vi "HandleObservationAsync.vi"(8 "error in (no error)":errorcluster, 10 "Acquisition.lvclass In":refnum<class "Acquisition.lvclass">, 11 "S4ACS_GUI in":refnum<class "S4GUI.lvclass">) -> (0 "error out":errorcluster, 2 "Acquisition.lvclass Out":refnum<class "Acquisition.lvclass">, 3 "S4ACS_GUI out":refnum<class "S4GUI.lvclass">)   [LabVIEW 2018, in "S4GUI.lvclass"]
uses:
  S4GUI.lvclass
  Acquisition/Acquisition.lvclass
  S4GUI.lvclass/S4GUI.ctl
  Instrument/Instrument.lvclass/Instrument.ctl
  Device/Optics/Optics.lvclass/Optics.ctl
  Server/Server.lvclass/Server.ctl
  Device/Optics/Opt_Selector/Opt_Selector.lvclass
  C:/Users/observer/Desktop/Sparc4GUI/SPARC4_GUI/Device/Optics/Optics.lvclass
  SyncBox/Sync Box.lvclass
  C:/Users/observer/Desktop/Sparc4GUI/SPARC4_GUI/Server/Server.lvclass
  Instrument/Instrument.lvclass
  StateMachine/State Machine.lvclass
  Trigger/Trigger.lvclass
  Channel/Channel.lvclass
  Device/Optics/Optics.lvclass
  Server/Server.lvclass
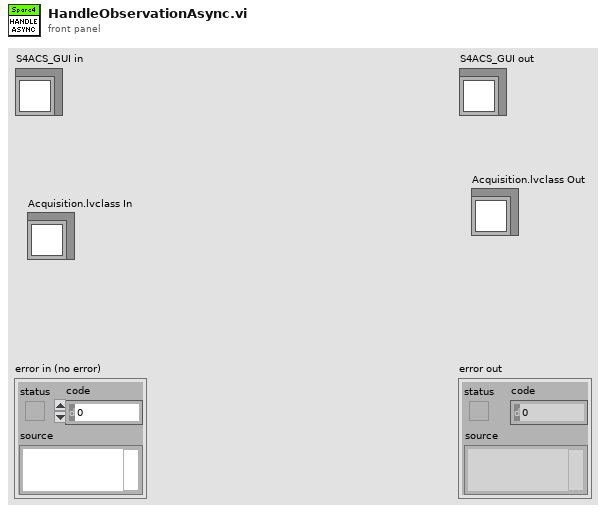
[diagram p1: front panel]
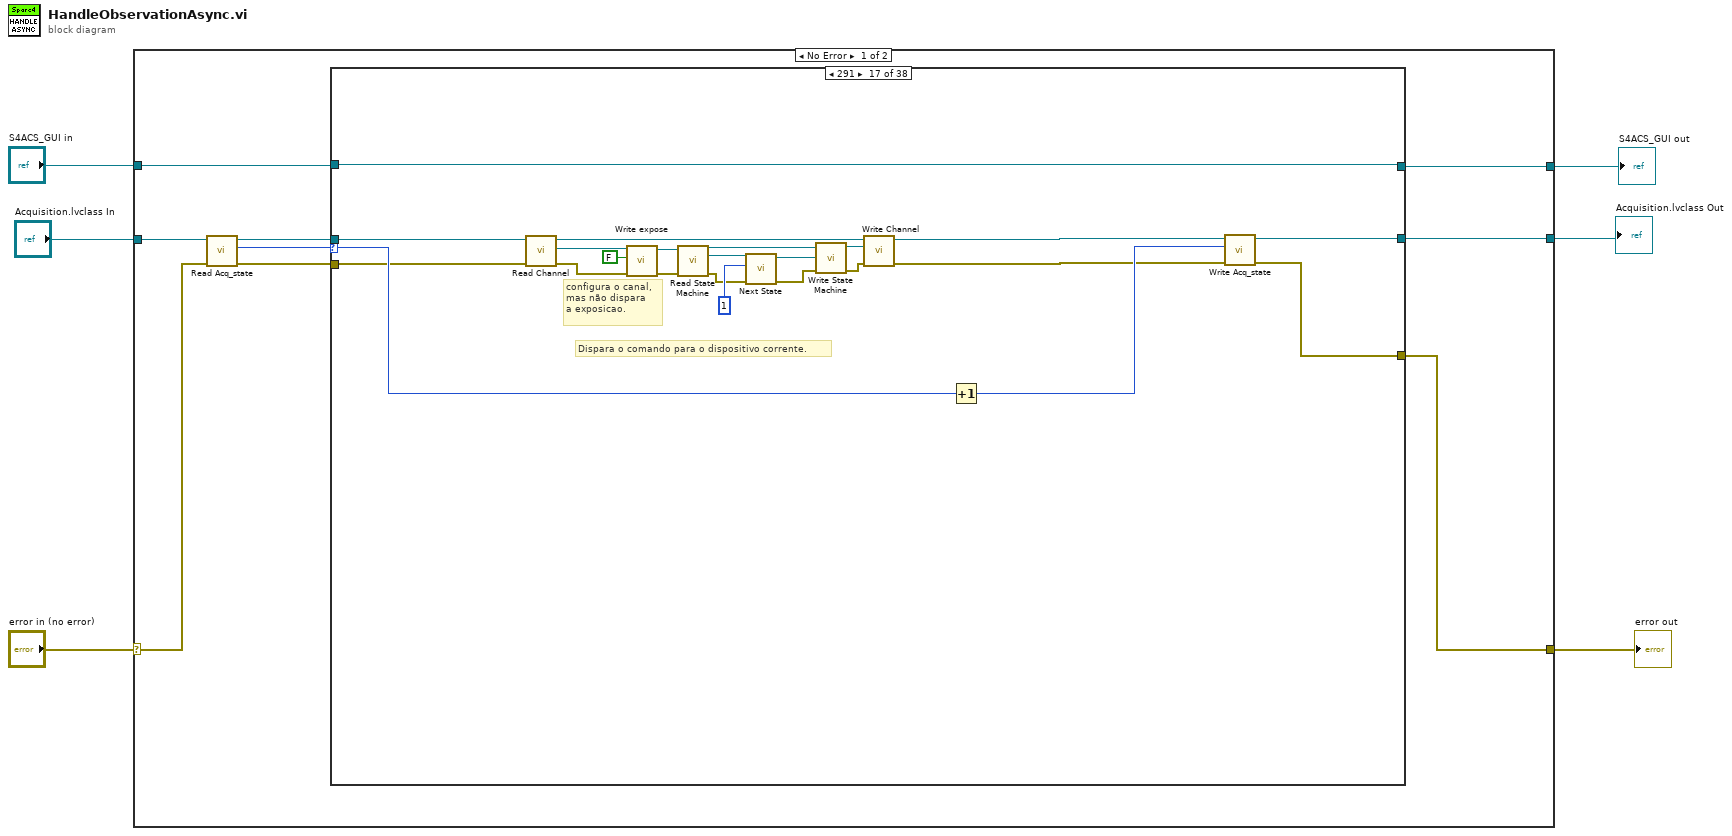
[diagram p0: block diagram]
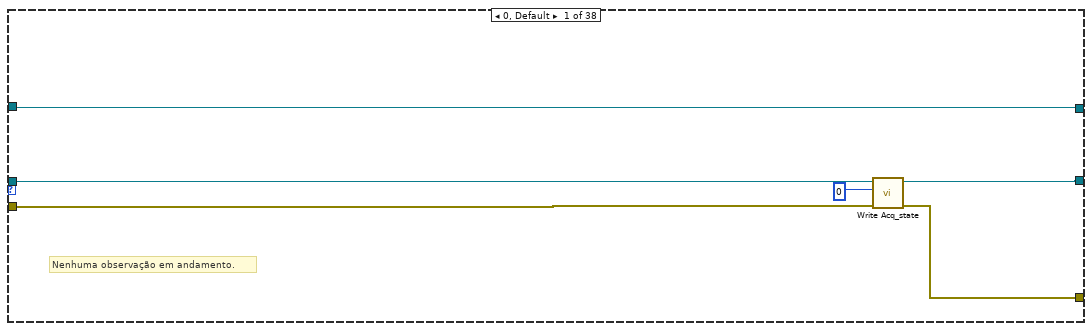
[diagram p2: hidden frame]
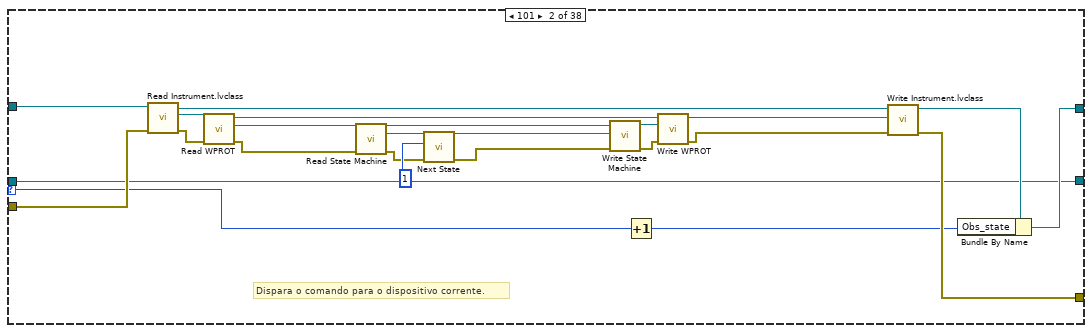
[diagram p3: hidden frame]
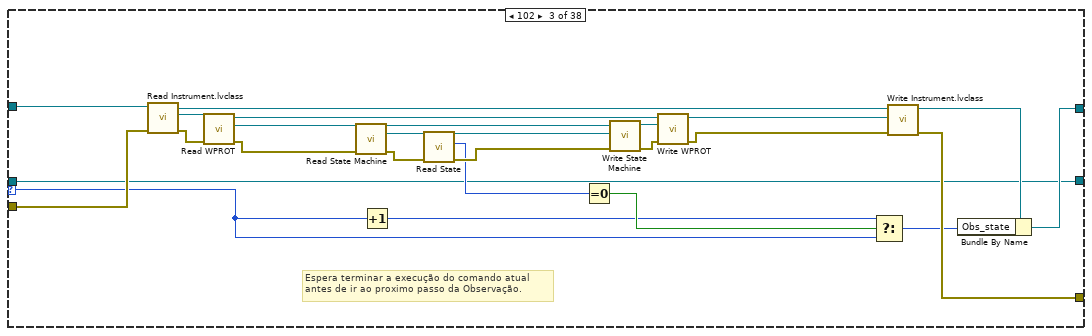
[diagram p4: hidden frame]
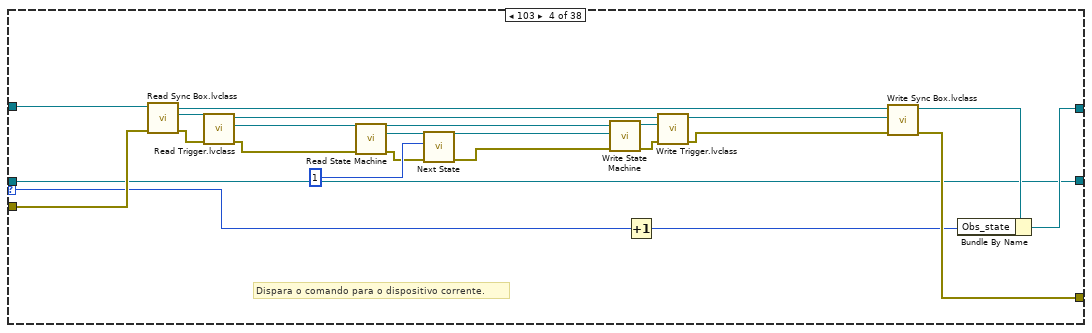
[diagram p5: hidden frame]
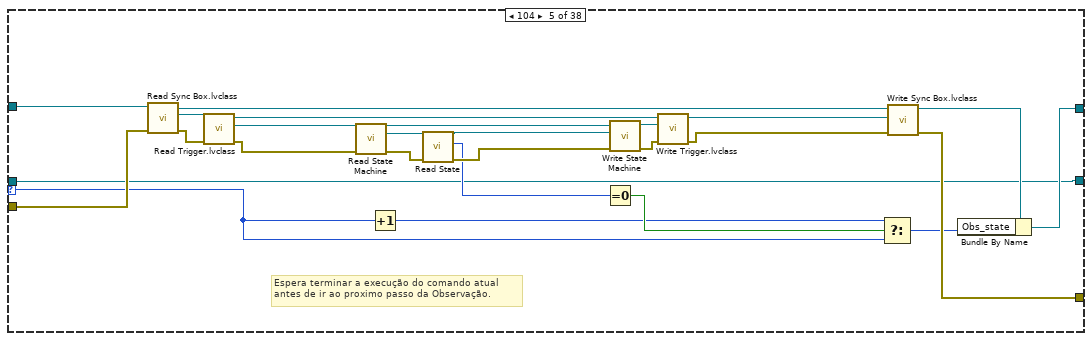
[diagram p6: hidden frame]
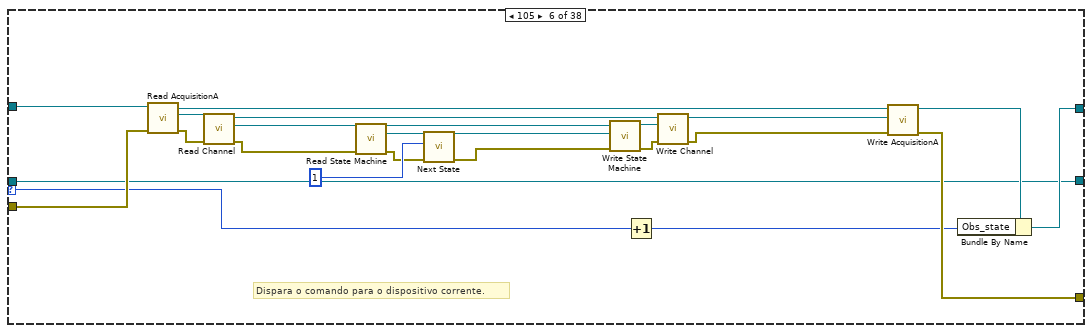
[diagram p7: hidden frame]
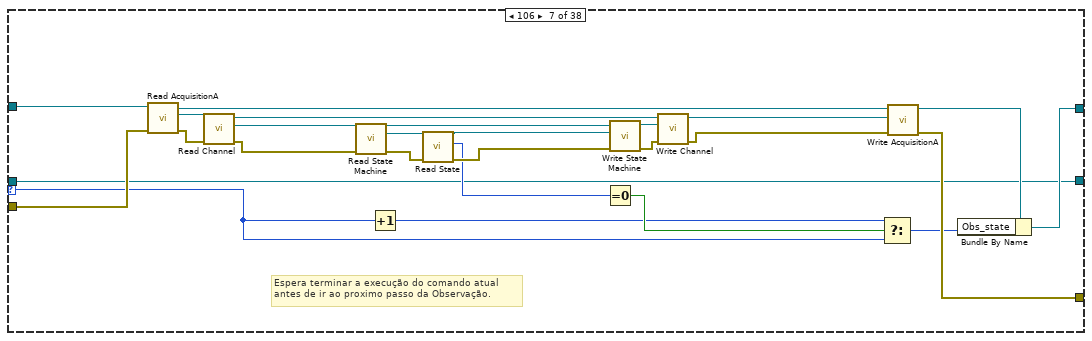
[diagram p8: hidden frame]
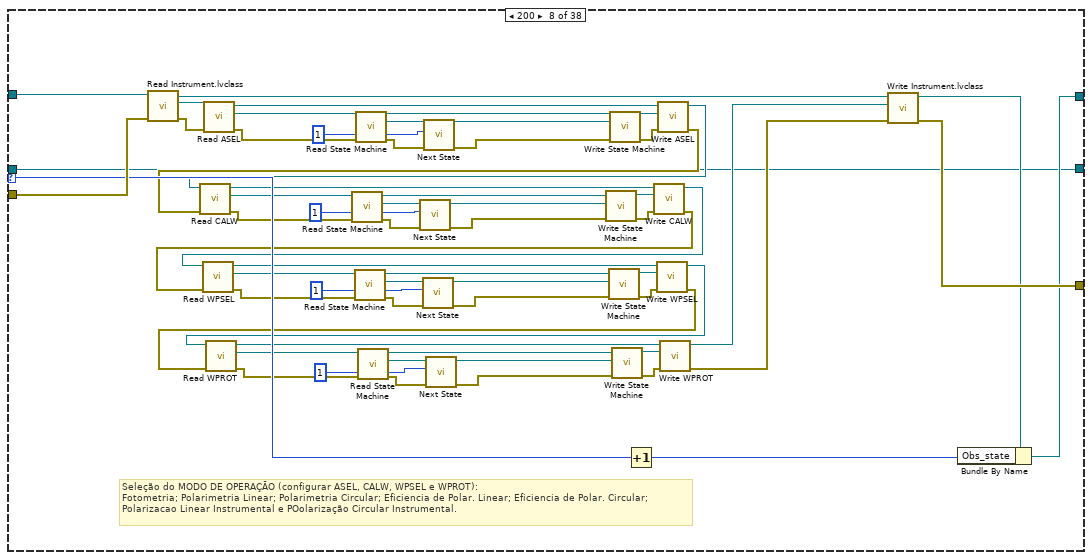
[diagram p9: hidden frame]
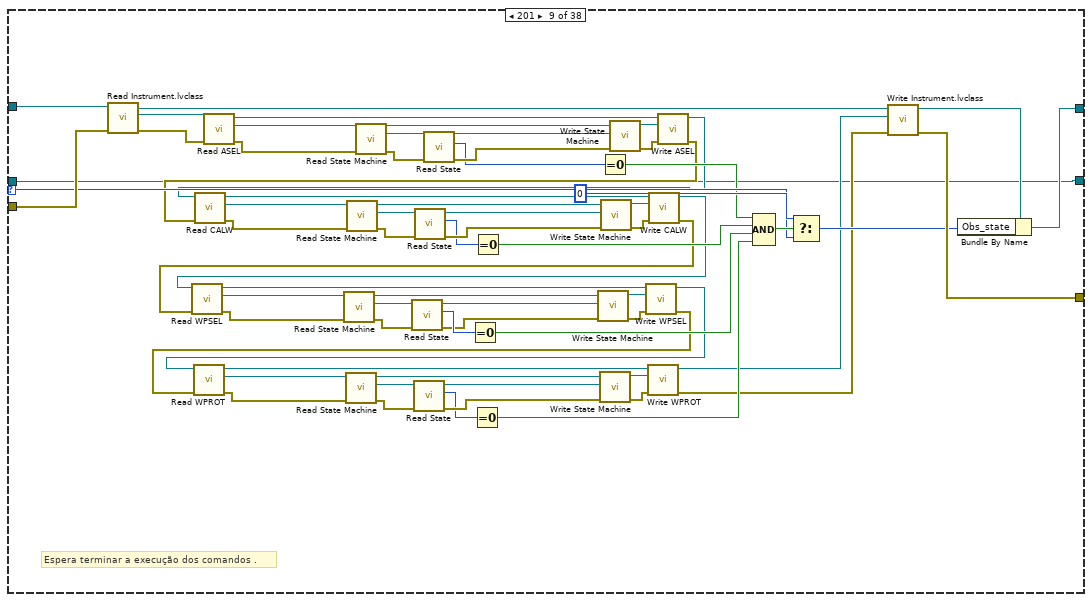
[diagram p10: hidden frame]
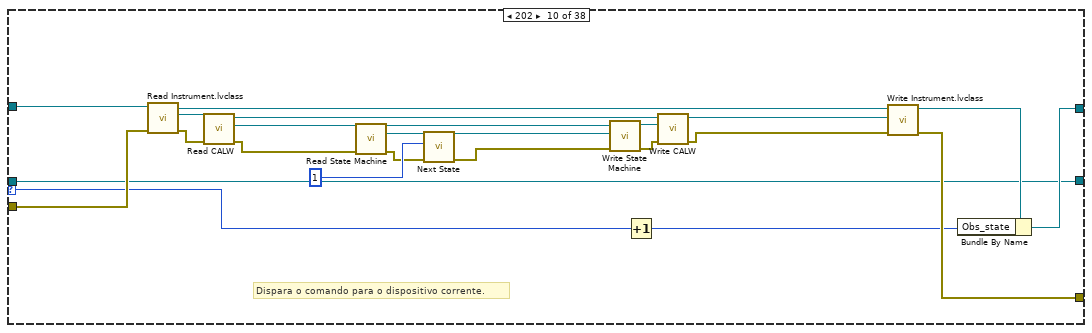
[diagram p11: hidden frame]
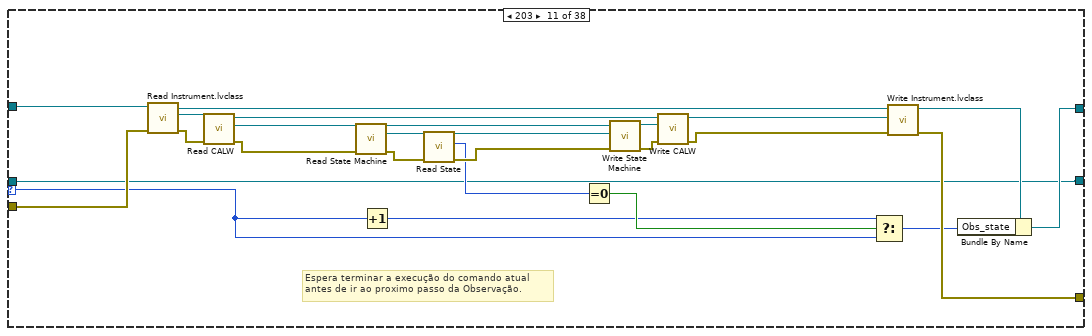
[diagram p12: hidden frame]
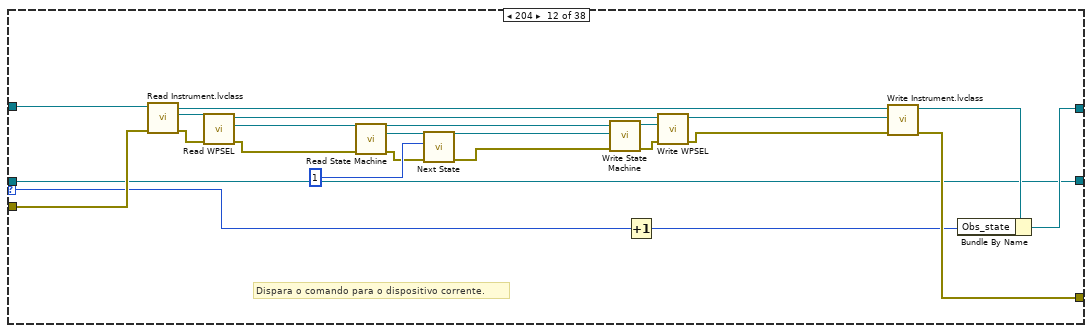
[diagram p13: hidden frame]
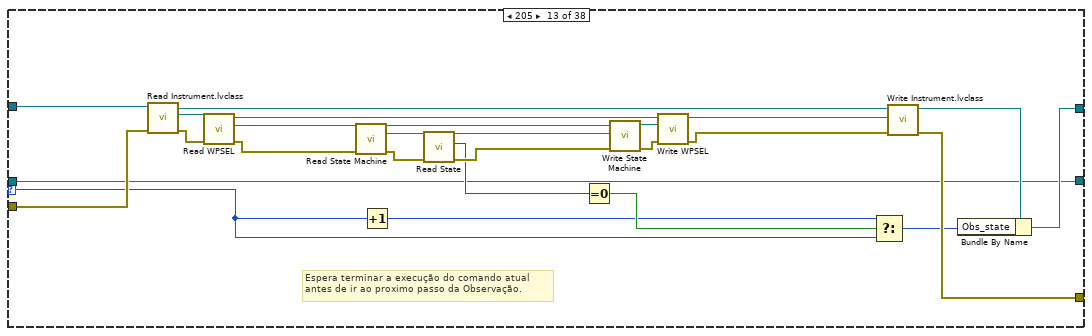
[diagram p14: hidden frame]
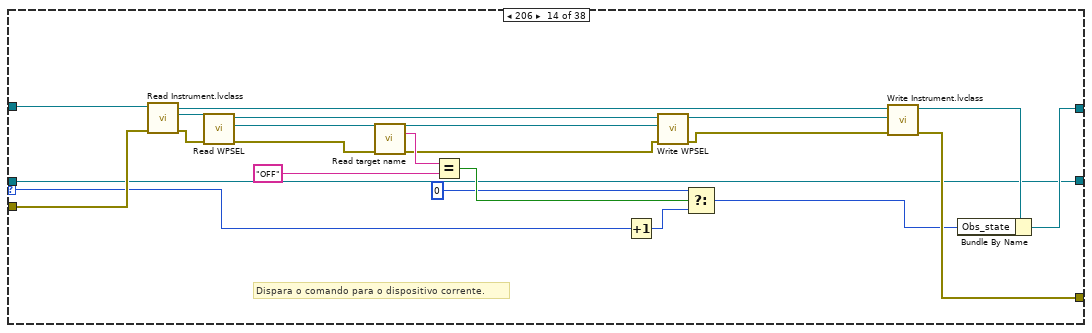
[diagram p15: hidden frame]
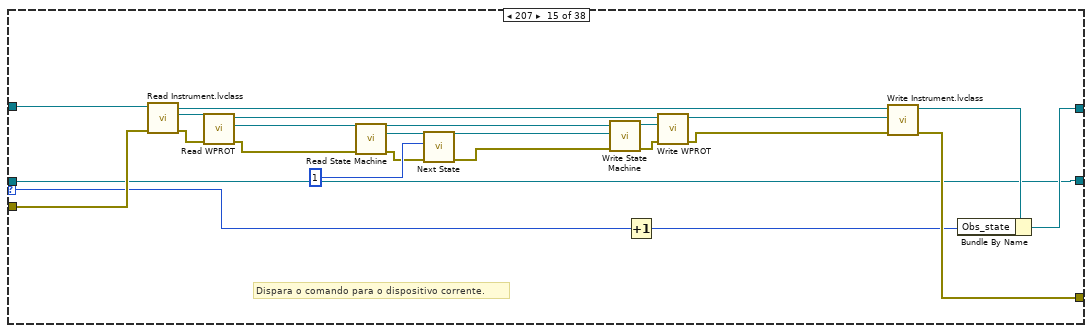
[diagram p16: hidden frame]
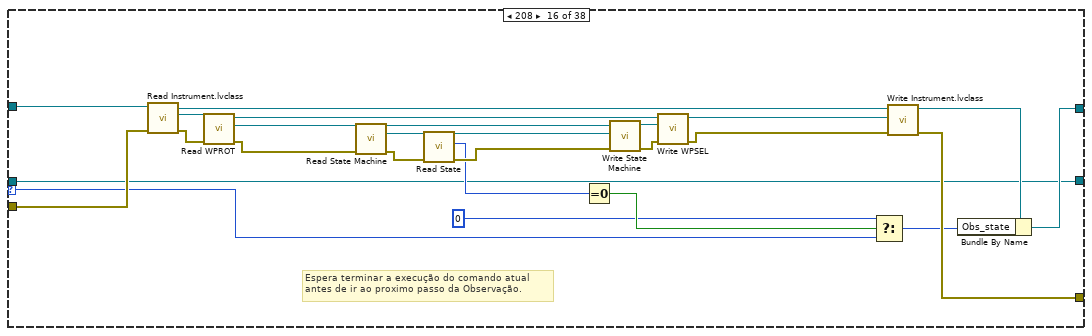
[diagram p17: hidden frame]
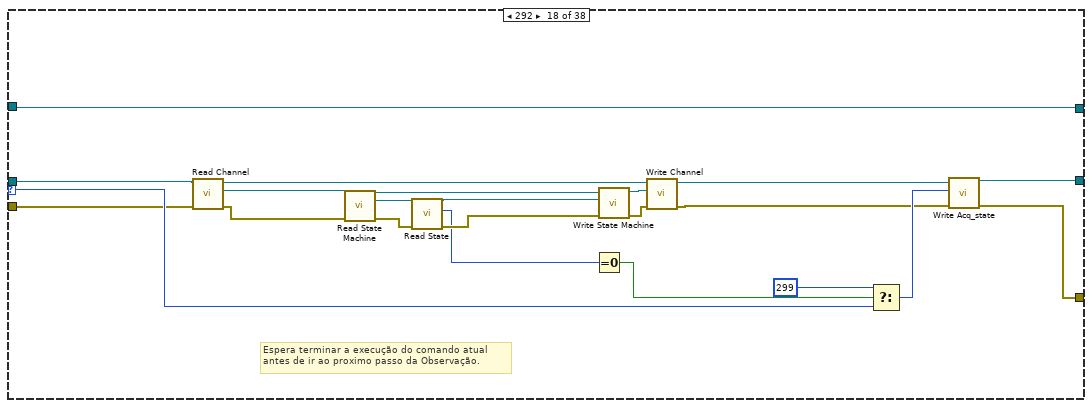
[diagram p18: hidden frame]
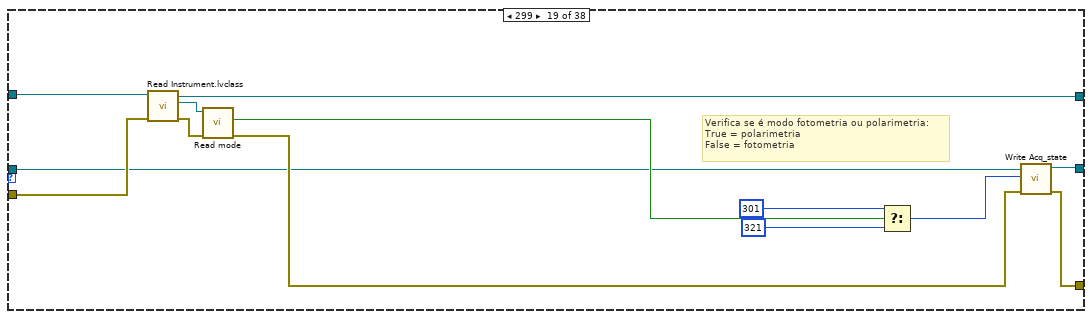
[diagram p19: hidden frame]
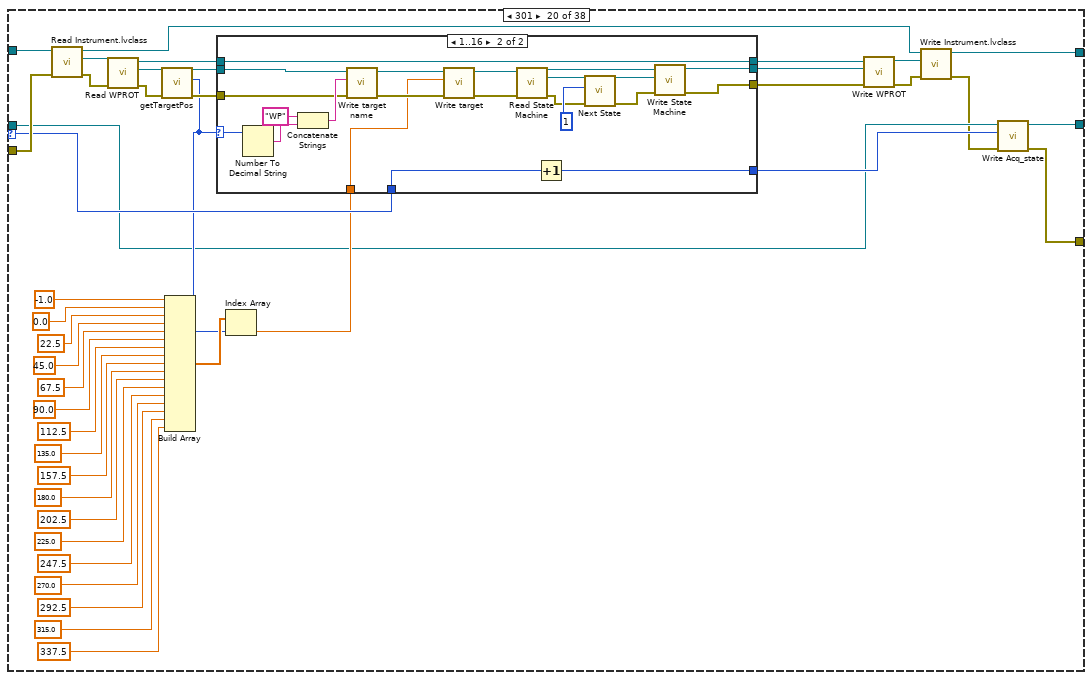
[diagram p20: hidden frame]
diagram:
  n1 = case shown="No Error" "error in (no error)" {
    selector: "error in (no error)" -> [w9 w1211]
    tunnel: [w15 w1211] -> w5
    tunnel: [w14 w1210] -> w3
    tunnel: "S4ACS_GUI in" -> [w13 w1210]
    tunnel: "Acquisition.lvclass In" -> [w12 w1209]
    tunnel: [w7 w1209] -> w1
    frame No Error {
      n2 = call-dynamic "Read Acq_state.vi"("error in (no error)"=w9, "Acquisition in"=w12) -> ("error out"=w8:errorcluster, "Acq_state"=w10:u32, "Acquisition out"=w11:refnum<class "Acquisition.lvclass">)  [unwired: 7 in]
      n3 = case shown="291" w10 {
        selector: w10 -> [_ w25 w48 w75 w98 w125 w148 w217 w281 w307 w330 w357 w380 w416 w430 w453 w492 w508 _ w570 w620 w644 w675 w732 w772 w788 w819 w873 w909 _ w959 w1016 w1056 w1077 w1131 w1167 _ _]
        tunnel: w13 -> [w20 w39 w65 w89 w115 w139 w165 w231 w299 w321 w347 w371 w397 w420 w444 w470 w479 w506 w534 w572 w631 w657 w677 w744 w763 w801 w821 w885 w902 w931 w961 w1028 w1044 w1079 w1143 w1160 w1191 w1208]
        tunnel: [w20 w23 w52 w73 w106 w123 w156 w215 w286 w305 w334 w355 w384 w415 w428 w457 w479 w506 w527 w537 w608 w643 w674 w726 w763 w787 w818 w872 w902 w931 w958 w1015 w1044 w1076 w1130 w1160 w1191 w1208] -> w14
        tunnel: w8 -> [w19 w38 w64 w88 w114 w138 w164 w230 w298 w320 w346 w370 w396 w419 w443 w469 w483 w500 w533 w571 w630 w656 w676 w743 w765 w800 w820 w884 w906 w938 w960 w1027 w1049 w1078 w1142 w1159 w1195 w1207]
        tunnel: [w16 w37 w63 w87 w113 w137 w163 w229 w297 w319 w345 w369 w395 w418 w442 w468 w477 w501 w523 w536 w610 w639 w670 w721 w759 w783 w813 w869 w900 w924 w953 w1012 w1043 w1073 w1127 w1163 w1181 w1207] -> w15
        tunnel: w11 -> [w18 w22 w46 w72 w96 w122 w146 w172 w235 w304 w328 w354 w378 w404 w427 w451 w484 w507 w524 w539 w612 w638 w669 w723 w766 w782 w814 w862 w907 w937 w954 w1011 w1050 w1071 w1120 w1158 w1196 w1206]
        tunnel: [w17 w22 w46 w72 w96 w122 w146 w172 w235 w304 w328 w354 w378 w404 w427 w451 w480 w502 w522 w535 w609 w640 w671 w722 w760 w786 w817 w870 w901 w925 w957 w1014 w1048 w1072 w1128 w1165 w1187 w1206] -> w7
        frame 0, Default {
          # "Nenhuma observação em andamento."
          n4 = call-dynamic "Write Acq_state.vi"("error in (no error)"=w19, "Acq_state"=u32 0 ("Obs_state"), "Acquisition in"=w18) -> ("error out"=w16:errorcluster, "Acquisition out"=w17:refnum<class "Acquisition.lvclass">)  [unwired: 7 in]
        }
        frame 101 {
          # "Dispara o comando para o dispositivo corrente."
          n5 = call "Read Instrument.lvclass.vi"("error in (no error)"=w38, "S4ACS_GUI in"=w39) -> ("error out"=w44:errorcluster, "Instrument.lvclass"=w45:refnum<class "Instrument.lvclass">, "S4ACS_GUI out"=w41:refnum<class "S4GUI.lvclass">)  [unwired: 7 in]
          n6 = call "Read WPROT.vi"("error in (no error)"=w44, "Instrument in"=w45) -> ("error out"=w31:errorcluster, "Opt_Selector.lvclass"=w30:refnum<class "Opt_Selector.lvclass">, "Instrument out"=w43:refnum<class "Instrument.lvclass">)  [unwired: 7 in]
          n7 = call-dynamic "Read State Machine.vi"("error in (no error)"=w31, "Device in"=w30) -> ("error out"=w34:errorcluster, "State Machine.lvclass"=w36:refnum<class "State Machine.lvclass">, "Device out"=w28:refnum<class "Opt_Selector.lvclass">)  [unwired: 7 in]
          n8 = call "Next State.vi"("error in (no error)"=w34, "New_State"=1, "State Machine in"=w36) -> ("error out"=w33:errorcluster, "State Machine out"=w32:refnum<class "State Machine.lvclass">)  [unwired: 7 in]
          n9 = call-dynamic "Write State Machine.vi"("error in (no error)"=w33, "State Machine.lvclass"=w32, "Device in"=w28) -> ("error out"=w27:errorcluster, "Device out"=w29:refnum<class "Opt_Selector.lvclass">)  [unwired: 7 in]
          n10 = Increment(x=w25) -> (x+1=w24:u32)
          n11 = call "Write WPROT.vi"("error in (no error)"=w27, "Opt_Selector.lvclass"=w29, "Instrument in"=w43) -> ("error out"=w40:errorcluster, "Instrument out"=w42:refnum<class "Instrument.lvclass">)  [unwired: 7 in]
          n12 = call "Write Instrument.lvclass.vi"("error in (no error)"=w40, "Instrument.lvclass"=w42, "S4ACS_GUI in"=w41) -> ("error out"=w37:errorcluster, "S4ACS_GUI out"=w26:refnum<class "S4GUI.lvclass">)  [unwired: 7 in]
          n13 = Bundle By Name(cluster=w26, "Obs_state"=w24) -> (w23:refnum<class "S4GUI.lvclass">)
        }
        frame 102 {
          # "Espera terminar a execução do comando atual \nantes de ir ao proximo passo da Observação."
          n14 = call "Read Instrument.lvclass.vi"("error in (no error)"=w64, "S4ACS_GUI in"=w65) -> ("error out"=w70:errorcluster, "Instrument.lvclass"=w71:refnum<class "Instrument.lvclass">, "S4ACS_GUI out"=w67:refnum<class "S4GUI.lvclass">)  [unwired: 7 in]
          n15 = call "Read WPROT.vi"("error in (no error)"=w70, "Instrument in"=w71) -> ("error out"=w58:errorcluster, "Opt_Selector.lvclass"=w57:refnum<class "Opt_Selector.lvclass">, "Instrument out"=w69:refnum<class "Instrument.lvclass">)  [unwired: 7 in]
          n16 = call-dynamic "Read State Machine.vi"("error in (no error)"=w58, "Device in"=w57) -> ("error out"=w61:errorcluster, "State Machine.lvclass"=w62:refnum<class "State Machine.lvclass">, "Device out"=w55:refnum<class "Opt_Selector.lvclass">)  [unwired: 7 in]
          n17 = Increment(x=w48) -> (x+1=w47:u32)
          n18 = call-dynamic "Read State.vi"("error in (no error)"=w61, "State Machine in"=w62) -> ("error out"=w60:errorcluster, "State"=w50:i32, "State Machine out"=w59:refnum<class "State Machine.lvclass">)  [unwired: 7 in]
          n19 = Equal To 0?(x=w50) -> (x = 0?=w51:bool)
          n20 = call-dynamic "Write State Machine.vi"("error in (no error)"=w60, "State Machine.lvclass"=w59, "Device in"=w55) -> ("error out"=w54:errorcluster, "Device out"=w56:refnum<class "Opt_Selector.lvclass">)  [unwired: 7 in]
          n21 = call "Write WPROT.vi"("error in (no error)"=w54, "Opt_Selector.lvclass"=w56, "Instrument in"=w69) -> ("error out"=w66:errorcluster, "Instrument out"=w68:refnum<class "Instrument.lvclass">)  [unwired: 7 in]
          n22 = Select(t=w47, s=w51, f=w48) -> (s? t:f=w49:u32)
          n23 = call "Write Instrument.lvclass.vi"("error in (no error)"=w66, "Instrument.lvclass"=w68, "S4ACS_GUI in"=w67) -> ("error out"=w63:errorcluster, "S4ACS_GUI out"=w53:refnum<class "S4GUI.lvclass">)  [unwired: 7 in]
          n24 = Bundle By Name(cluster=w53, "Obs_state"=w49) -> (w52:refnum<class "S4GUI.lvclass">)
        }
        frame 103 {
          # "Dispara o comando para o dispositivo corrente."
          n25 = call-dynamic "Read Sync Box.lvclass.vi"("error in (no error)"=w88, "SPARC4_AC in"=w89) -> ("error out"=w94:errorcluster, "Sync Box.lvclass"=w95:refnum<class "Sync Box.lvclass">, "SPARC4_AC out"=w91:refnum<class "S4GUI.lvclass">)  [unwired: 7 in]
          n26 = call-dynamic "Read Trigger.lvclass.vi"("error in (no error)"=w94, "Sync Box in"=w95) -> ("error out"=w81:errorcluster, "Trigger.lvclass"=w80:refnum<class "Trigger.lvclass">, "Sync Box out"=w93:refnum<class "Sync Box.lvclass">)  [unwired: 7 in]
          n27 = call-dynamic "Read State Machine.vi"("error in (no error)"=w81, "Device in"=w80) -> ("error out"=w84:errorcluster, "State Machine.lvclass"=w86:refnum<class "State Machine.lvclass">, "Device out"=w78:refnum<class "Trigger.lvclass">)  [unwired: 7 in]
          n28 = call "Next State.vi"("error in (no error)"=w84, "New_State"=1, "State Machine in"=w86) -> ("error out"=w83:errorcluster, "State Machine out"=w82:refnum<class "State Machine.lvclass">)  [unwired: 7 in]
          n29 = call-dynamic "Write State Machine.vi"("error in (no error)"=w83, "State Machine.lvclass"=w82, "Device in"=w78) -> ("error out"=w77:errorcluster, "Device out"=w79:refnum<class "Trigger.lvclass">)  [unwired: 7 in]
          n30 = Increment(x=w75) -> (x+1=w74:u32)
          n31 = call-dynamic "Write Trigger.lvclass.vi"("error in (no error)"=w77, "Trigger.lvclass"=w79, "Sync Box in"=w93) -> ("error out"=w90:errorcluster, "Sync Box out"=w92:refnum<class "Sync Box.lvclass">)  [unwired: 7 in]
          n32 = call-dynamic "Write Sync Box.lvclass.vi"("error in (no error)"=w90, "Sync Box.lvclass"=w92, "SPARC4_AC in"=w91) -> ("error out"=w87:errorcluster, "SPARC4_AC out"=w76:refnum<class "S4GUI.lvclass">)  [unwired: 7 in]
          n33 = Bundle By Name(cluster=w76, "Obs_state"=w74) -> (w73:refnum<class "S4GUI.lvclass">)
        }
        frame 104 {
          # "Espera terminar a execução do comando atual \nantes de ir ao proximo passo da Observação."
          n34 = call-dynamic "Read Sync Box.lvclass.vi"("error in (no error)"=w114, "SPARC4_AC in"=w115) -> ("error out"=w120:errorcluster, "Sync Box.lvclass"=w121:refnum<class "Sync Box.lvclass">, "SPARC4_AC out"=w117:refnum<class "S4GUI.lvclass">)  [unwired: 7 in]
          n35 = call-dynamic "Read Trigger.lvclass.vi"("error in (no error)"=w120, "Sync Box in"=w121) -> ("error out"=w112:errorcluster, "Trigger.lvclass"=w111:refnum<class "Trigger.lvclass">, "Sync Box out"=w119:refnum<class "Sync Box.lvclass">)  [unwired: 7 in]
          n36 = call-dynamic "Read State Machine.vi"("error in (no error)"=w112, "Device in"=w111) -> ("error out"=w103:errorcluster, "State Machine.lvclass"=w105:refnum<class "State Machine.lvclass">, "Device out"=w109:refnum<class "Trigger.lvclass">)  [unwired: 7 in]
          n37 = Increment(x=w98) -> (x+1=w100:u32)
          n38 = call-dynamic "Read State.vi"("error in (no error)"=w103, "State Machine in"=w105) -> ("error out"=w102:errorcluster, "State"=w97:i32, "State Machine out"=w104:refnum<class "State Machine.lvclass">)  [unwired: 7 in]
          n39 = Equal To 0?(x=w97) -> (x = 0?=w101:bool)
          n40 = call-dynamic "Write State Machine.vi"("error in (no error)"=w102, "State Machine.lvclass"=w104, "Device in"=w109) -> ("error out"=w108:errorcluster, "Device out"=w110:refnum<class "Trigger.lvclass">)  [unwired: 7 in]
          n41 = call-dynamic "Write Trigger.lvclass.vi"("error in (no error)"=w108, "Trigger.lvclass"=w110, "Sync Box in"=w119) -> ("error out"=w116:errorcluster, "Sync Box out"=w118:refnum<class "Sync Box.lvclass">)  [unwired: 7 in]
          n42 = Select(t=w100, s=w101, f=w98) -> (s? t:f=w99:u32)
          n43 = call-dynamic "Write Sync Box.lvclass.vi"("error in (no error)"=w116, "Sync Box.lvclass"=w118, "SPARC4_AC in"=w117) -> ("error out"=w113:errorcluster, "SPARC4_AC out"=w107:refnum<class "S4GUI.lvclass">)  [unwired: 7 in]
          n44 = Bundle By Name(cluster=w107, "Obs_state"=w99) -> (w106:refnum<class "S4GUI.lvclass">)
        }
        frame 105 {
          # "Dispara o comando para o dispositivo corrente."
          n45 = call-dynamic "Read AcquisitionA.vi"("error in (no error)"=w138, "S4ACS_GUI in"=w139) -> ("error out"=w144:errorcluster, "Acquisition.lvclass"=w145:refnum<class "Acquisition.lvclass">, "S4ACS_GUI out"=w141:refnum<class "S4GUI.lvclass">)  [unwired: 7 in]
          n46 = call-dynamic "Read Channel.vi"("error in (no error)"=w144, "Acquisition in"=w145) -> ("error out"=w131:errorcluster, "Channel.lvclass"=w130:refnum<class "Channel.lvclass">, "Acquisition out"=w143:refnum<class "Acquisition.lvclass">)  [unwired: 7 in]
          n47 = call-dynamic "Read State Machine.vi"("error in (no error)"=w131, "Device in"=w130) -> ("error out"=w134:errorcluster, "State Machine.lvclass"=w136:refnum<class "State Machine.lvclass">, "Device out"=w128:refnum<class "Channel.lvclass">)  [unwired: 7 in]
          n48 = call "Next State.vi"("error in (no error)"=w134, "New_State"=1, "State Machine in"=w136) -> ("error out"=w133:errorcluster, "State Machine out"=w132:refnum<class "State Machine.lvclass">)  [unwired: 7 in]
          n49 = call-dynamic "Write State Machine.vi"("error in (no error)"=w133, "State Machine.lvclass"=w132, "Device in"=w128) -> ("error out"=w127:errorcluster, "Device out"=w129:refnum<class "Channel.lvclass">)  [unwired: 7 in]
          n50 = Increment(x=w125) -> (x+1=w124:u32)
          n51 = call-dynamic "Write Channel.vi"("error in (no error)"=w127, "Channel.lvclass"=w129, "Acquisition in"=w143) -> ("error out"=w140:errorcluster, "Acquisition out"=w142:refnum<class "Acquisition.lvclass">)  [unwired: 7 in]
          n52 = call-dynamic "Write AcquisitionA.vi"("error in (no error)"=w140, "Acquisition.lvclass"=w142, "S4ACS_GUI in"=w141) -> ("error out"=w137:errorcluster, "S4ACS_GUI out"=w126:refnum<class "S4GUI.lvclass">)  [unwired: 7 in]
          n53 = Bundle By Name(cluster=w126, "Obs_state"=w124) -> (w123:refnum<class "S4GUI.lvclass">)
        }
        frame 106 {
          # "Espera terminar a execução do comando atual \nantes de ir ao proximo passo da Observação."
          n54 = call-dynamic "Read AcquisitionA.vi"("error in (no error)"=w164, "S4ACS_GUI in"=w165) -> ("error out"=w170:errorcluster, "Acquisition.lvclass"=w171:refnum<class "Acquisition.lvclass">, "S4ACS_GUI out"=w167:refnum<class "S4GUI.lvclass">)  [unwired: 7 in]
          n55 = call-dynamic "Read Channel.vi"("error in (no error)"=w170, "Acquisition in"=w171) -> ("error out"=w162:errorcluster, "Channel.lvclass"=w161:refnum<class "Channel.lvclass">, "Acquisition out"=w169:refnum<class "Acquisition.lvclass">)  [unwired: 7 in]
          n56 = call-dynamic "Read State Machine.vi"("error in (no error)"=w162, "Device in"=w161) -> ("error out"=w153:errorcluster, "State Machine.lvclass"=w155:refnum<class "State Machine.lvclass">, "Device out"=w159:refnum<class "Channel.lvclass">)  [unwired: 7 in]
          n57 = Increment(x=w148) -> (x+1=w150:u32)
          n58 = call-dynamic "Read State.vi"("error in (no error)"=w153, "State Machine in"=w155) -> ("error out"=w152:errorcluster, "State"=w147:i32, "State Machine out"=w154:refnum<class "State Machine.lvclass">)  [unwired: 7 in]
          n59 = Equal To 0?(x=w147) -> (x = 0?=w151:bool)
          n60 = call-dynamic "Write State Machine.vi"("error in (no error)"=w152, "State Machine.lvclass"=w154, "Device in"=w159) -> ("error out"=w158:errorcluster, "Device out"=w160:refnum<class "Channel.lvclass">)  [unwired: 7 in]
          n61 = call-dynamic "Write Channel.vi"("error in (no error)"=w158, "Channel.lvclass"=w160, "Acquisition in"=w169) -> ("error out"=w166:errorcluster, "Acquisition out"=w168:refnum<class "Acquisition.lvclass">)  [unwired: 7 in]
          n62 = Select(t=w150, s=w151, f=w148) -> (s? t:f=w149:u32)
          n63 = call-dynamic "Write AcquisitionA.vi"("error in (no error)"=w166, "Acquisition.lvclass"=w168, "S4ACS_GUI in"=w167) -> ("error out"=w163:errorcluster, "S4ACS_GUI out"=w157:refnum<class "S4GUI.lvclass">)  [unwired: 7 in]
          n64 = Bundle By Name(cluster=w157, "Obs_state"=w149) -> (w156:refnum<class "S4GUI.lvclass">)
        }
        frame 200 {
          # "Seleção do MODO DE OPERAÇÃO (configurar ASEL, CALW, WPSEL e WPROT): \nFotometria; Polarimetria Linear; Polarimetria Circular; Eficiencia de Polar. Linear; Eficiencia de Polar. Circular;\nPolarizacao Linear Instrumental e POolarização Circular Instrumental."
          n65 = call "Read Instrument.lvclass.vi"("error in (no error)"=w230, "S4ACS_GUI in"=w231) -> ("error out"=w234:errorcluster, "Instrument.lvclass"=w194:refnum<class "Instrument.lvclass">, "S4ACS_GUI out"=w232:refnum<class "S4GUI.lvclass">)  [unwired: 7 in]
          n66 = call "Read ASEL.vi"("error in (no error)"=w234, "Instrument in"=w194) -> ("error out"=w223:errorcluster, "Opt_Selector.lvclass"=w222:refnum<class "Opt_Selector.lvclass">, "Instrument out"=w233:refnum<class "Instrument.lvclass">)  [unwired: 7 in]
          n67 = call-dynamic "Read State Machine.vi"("error in (no error)"=w223, "Device in"=w222) -> ("error out"=w226:errorcluster, "State Machine.lvclass"=w228:refnum<class "State Machine.lvclass">, "Device out"=w220:refnum<class "Opt_Selector.lvclass">)  [unwired: 7 in]
          n68 = call "Next State.vi"("error in (no error)"=w226, "New_State"=1, "State Machine in"=w228) -> ("error out"=w225:errorcluster, "State Machine out"=w224:refnum<class "State Machine.lvclass">)  [unwired: 7 in]
          n69 = call-dynamic "Write State Machine.vi"("error in (no error)"=w225, "State Machine.lvclass"=w224, "Device in"=w220) -> ("error out"=w219:errorcluster, "Device out"=w221:refnum<class "Opt_Selector.lvclass">)  [unwired: 7 in]
          n70 = Increment(x=w217) -> (x+1=w216:u32)
          n71 = call "Write ASEL.vi"("error in (no error)"=w219, "Opt_Selector.lvclass"=w221, "Instrument in"=w233) -> ("error out"=w175:errorcluster, "Instrument out"=w193:refnum<class "Instrument.lvclass">)  [unwired: 7 in]
          n72 = call "Read CALW.vi"("error in (no error)"=w175, "Instrument in"=w193) -> ("error out"=w210:errorcluster, "Opt_Selector.lvclass"=w211:refnum<class "Opt_Selector.lvclass">, "Instrument out"=w192:refnum<class "Instrument.lvclass">)  [unwired: 7 in]
          n73 = call-dynamic "Read State Machine.vi"("error in (no error)"=w210, "Device in"=w211) -> ("error out"=w207:errorcluster, "State Machine.lvclass"=w205:refnum<class "State Machine.lvclass">, "Device out"=w213:refnum<class "Opt_Selector.lvclass">)  [unwired: 7 in]
          n74 = call "Next State.vi"("error in (no error)"=w207, "New_State"=1, "State Machine in"=w205) -> ("error out"=w208:errorcluster, "State Machine out"=w209:refnum<class "State Machine.lvclass">)  [unwired: 7 in]
          n75 = call-dynamic "Write State Machine.vi"("error in (no error)"=w208, "State Machine.lvclass"=w209, "Device in"=w213) -> ("error out"=w214:errorcluster, "Device out"=w212:refnum<class "Opt_Selector.lvclass">)  [unwired: 7 in]
          n76 = call "Write CALW.vi"("error in (no error)"=w214, "Opt_Selector.lvclass"=w212, "Instrument in"=w192) -> ("error out"=w174:errorcluster, "Instrument out"=w191:refnum<class "Instrument.lvclass">)  [unwired: 7 in]
          n77 = call "Read WPSEL.vi"("error in (no error)"=w174, "Instrument in"=w191) -> ("error out"=w199:errorcluster, "Opt_Selector.lvclass"=w198:refnum<class "Opt_Selector.lvclass">, "Instrument out"=w190:refnum<class "Instrument.lvclass">)  [unwired: 7 in]
          n78 = call-dynamic "Read State Machine.vi"("error in (no error)"=w199, "Device in"=w198) -> ("error out"=w202:errorcluster, "State Machine.lvclass"=w204:refnum<class "State Machine.lvclass">, "Device out"=w196:refnum<class "Opt_Selector.lvclass">)  [unwired: 7 in]
          n79 = call "Next State.vi"("error in (no error)"=w202, "New_State"=1, "State Machine in"=w204) -> ("error out"=w201:errorcluster, "State Machine out"=w200:refnum<class "State Machine.lvclass">)  [unwired: 7 in]
          n80 = call-dynamic "Write State Machine.vi"("error in (no error)"=w201, "State Machine.lvclass"=w200, "Device in"=w196) -> ("error out"=w195:errorcluster, "Device out"=w197:refnum<class "Opt_Selector.lvclass">)  [unwired: 7 in]
          n81 = call "Write WPSEL.vi"("error in (no error)"=w195, "Opt_Selector.lvclass"=w197, "Instrument in"=w190) -> ("error out"=w173:errorcluster, "Instrument out"=w179:refnum<class "Instrument.lvclass">)  [unwired: 7 in]
          n82 = call "Read WPROT.vi"("error in (no error)"=w173, "Instrument in"=w179) -> ("error out"=w185:errorcluster, "Opt_Selector.lvclass"=w186:refnum<class "Opt_Selector.lvclass">, "Instrument out"=w178:refnum<class "Instrument.lvclass">)  [unwired: 7 in]
          n83 = call-dynamic "Read State Machine.vi"("error in (no error)"=w185, "Device in"=w186) -> ("error out"=w182:errorcluster, "State Machine.lvclass"=w180:refnum<class "State Machine.lvclass">, "Device out"=w188:refnum<class "Opt_Selector.lvclass">)  [unwired: 7 in]
          n84 = call "Next State.vi"("error in (no error)"=w182, "New_State"=1, "State Machine in"=w180) -> ("error out"=w183:errorcluster, "State Machine out"=w184:refnum<class "State Machine.lvclass">)  [unwired: 7 in]
          n85 = call-dynamic "Write State Machine.vi"("error in (no error)"=w183, "State Machine.lvclass"=w184, "Device in"=w188) -> ("error out"=w189:errorcluster, "Device out"=w187:refnum<class "Opt_Selector.lvclass">)  [unwired: 7 in]
          n86 = call "Write WPROT.vi"("error in (no error)"=w189, "Opt_Selector.lvclass"=w187, "Instrument in"=w178) -> ("error out"=w176:errorcluster, "Instrument out"=w177:refnum<class "Instrument.lvclass">)  [unwired: 7 in]
          n87 = call "Write Instrument.lvclass.vi"("error in (no error)"=w176, "Instrument.lvclass"=w177, "S4ACS_GUI in"=w232) -> ("error out"=w229:errorcluster, "S4ACS_GUI out"=w218:refnum<class "S4GUI.lvclass">)  [unwired: 7 in]
          n88 = Bundle By Name(cluster=w218, "Obs_state"=w216) -> (w215:refnum<class "S4GUI.lvclass">)
        }
        frame 201 {
          # "Espera terminar a execução dos comandos ."
          n89 = call "Read Instrument.lvclass.vi"("error in (no error)"=w298, "S4ACS_GUI in"=w299) -> ("error out"=w302:errorcluster, "Instrument.lvclass"=w303:refnum<class "Instrument.lvclass">, "S4ACS_GUI out"=w300:refnum<class "S4GUI.lvclass">)  [unwired: 7 in]
          n90 = call "Read ASEL.vi"("error in (no error)"=w302, "Instrument in"=w303) -> ("error out"=w292:errorcluster, "Opt_Selector.lvclass"=w291:refnum<class "Opt_Selector.lvclass">, "Instrument out"=w301:refnum<class "Instrument.lvclass">)  [unwired: 7 in]
          n91 = call-dynamic "Read State Machine.vi"("error in (no error)"=w292, "Device in"=w291) -> ("error out"=w295:errorcluster, "State Machine.lvclass"=w296:refnum<class "State Machine.lvclass">, "Device out"=w289:refnum<class "Opt_Selector.lvclass">)  [unwired: 7 in]
          n92 = call-dynamic "Read State.vi"("error in (no error)"=w295, "State Machine in"=w296) -> ("error out"=w294:errorcluster, "State"=w285:i32, "State Machine out"=w293:refnum<class "State Machine.lvclass">)  [unwired: 7 in]
          n93 = Equal To 0?(x=w285) -> (x = 0?=w280:bool)
          n94 = call-dynamic "Write State Machine.vi"("error in (no error)"=w294, "State Machine.lvclass"=w293, "Device in"=w289) -> ("error out"=w288:errorcluster, "Device out"=w290:refnum<class "Opt_Selector.lvclass">)  [unwired: 7 in]
          n95 = call "Write ASEL.vi"("error in (no error)"=w288, "Opt_Selector.lvclass"=w290, "Instrument in"=w301) -> ("error out"=w242:errorcluster, "Instrument out"=w243:refnum<class "Instrument.lvclass">)  [unwired: 7 in]
          n96 = call "Read CALW.vi"("error in (no error)"=w242, "Instrument in"=w243) -> ("error out"=w275:errorcluster, "Opt_Selector.lvclass"=w276:refnum<class "Opt_Selector.lvclass">, "Instrument out"=w246:refnum<class "Instrument.lvclass">)  [unwired: 7 in]
          n97 = call-dynamic "Read State Machine.vi"("error in (no error)"=w275, "Device in"=w276) -> ("error out"=w272:errorcluster, "State Machine.lvclass"=w271:refnum<class "State Machine.lvclass">, "Device out"=w278:refnum<class "Opt_Selector.lvclass">)  [unwired: 7 in]
          n98 = call-dynamic "Read State.vi"("error in (no error)"=w272, "State Machine in"=w271) -> ("error out"=w273:errorcluster, "State"=w270:i32, "State Machine out"=w274:refnum<class "State Machine.lvclass">)  [unwired: 7 in]
          n99 = Equal To 0?(x=w270) -> (x = 0?=w269:bool)
          n100 = call-dynamic "Write State Machine.vi"("error in (no error)"=w273, "State Machine.lvclass"=w274, "Device in"=w278) -> ("error out"=w279:errorcluster, "Device out"=w277:refnum<class "Opt_Selector.lvclass">)  [unwired: 7 in]
          n101 = call "Write CALW.vi"("error in (no error)"=w279, "Opt_Selector.lvclass"=w277, "Instrument in"=w246) -> ("error out"=w240:errorcluster, "Instrument out"=w241:refnum<class "Instrument.lvclass">)  [unwired: 7 in]
          n102 = call "Read WPSEL.vi"("error in (no error)"=w240, "Instrument in"=w241) -> ("error out"=w263:errorcluster, "Opt_Selector.lvclass"=w262:refnum<class "Opt_Selector.lvclass">, "Instrument out"=w245:refnum<class "Instrument.lvclass">)  [unwired: 7 in]
          n103 = call-dynamic "Read State Machine.vi"("error in (no error)"=w263, "Device in"=w262) -> ("error out"=w266:errorcluster, "State Machine.lvclass"=w267:refnum<class "State Machine.lvclass">, "Device out"=w260:refnum<class "Opt_Selector.lvclass">)  [unwired: 7 in]
          n104 = call-dynamic "Read State.vi"("error in (no error)"=w266, "State Machine in"=w267) -> ("error out"=w265:errorcluster, "State"=w268:i32, "State Machine out"=w264:refnum<class "State Machine.lvclass">)  [unwired: 7 in]
          n105 = Equal To 0?(x=w268) -> (x = 0?=w248:bool)
          n106 = call-dynamic "Write State Machine.vi"("error in (no error)"=w265, "State Machine.lvclass"=w264, "Device in"=w260) -> ("error out"=w259:errorcluster, "Device out"=w261:refnum<class "Opt_Selector.lvclass">)  [unwired: 7 in]
          n107 = call "Write WPSEL.vi"("error in (no error)"=w259, "Opt_Selector.lvclass"=w261, "Instrument in"=w245) -> ("error out"=w238:errorcluster, "Instrument out"=w239:refnum<class "Instrument.lvclass">)  [unwired: 7 in]
          n108 = call "Read WPROT.vi"("error in (no error)"=w238, "Instrument in"=w239) -> ("error out"=w254:errorcluster, "Opt_Selector.lvclass"=w255:refnum<class "Opt_Selector.lvclass">, "Instrument out"=w244:refnum<class "Instrument.lvclass">)  [unwired: 7 in]
          n109 = call-dynamic "Read State Machine.vi"("error in (no error)"=w254, "Device in"=w255) -> ("error out"=w251:errorcluster, "State Machine.lvclass"=w250:refnum<class "State Machine.lvclass">, "Device out"=w257:refnum<class "Opt_Selector.lvclass">)  [unwired: 7 in]
          n110 = call-dynamic "Read State.vi"("error in (no error)"=w251, "State Machine in"=w250) -> ("error out"=w252:errorcluster, "State"=w249:i32, "State Machine out"=w253:refnum<class "State Machine.lvclass">)  [unwired: 7 in]
          n111 = Equal To 0?(x=w249) -> (x = 0?=w247:bool)
          n112 = call-dynamic "Write State Machine.vi"("error in (no error)"=w252, "State Machine.lvclass"=w253, "Device in"=w257) -> ("error out"=w258:errorcluster, "Device out"=w256:refnum<class "Opt_Selector.lvclass">)  [unwired: 7 in]
          n113 = call "Write WPROT.vi"("error in (no error)"=w258, "Opt_Selector.lvclass"=w256, "Instrument in"=w244) -> ("error out"=w236:errorcluster, "Instrument out"=w237:refnum<class "Instrument.lvclass">)  [unwired: 7 in]
          n114 = Compound Arithmetic op=AND(w280, w269, w248, w247) -> (w282:bool)
          n115 = Select(t=u32 0, s=w282, f=w281) -> (s? t:f=w284:u32)
          n116 = call "Write Instrument.lvclass.vi"("error in (no error)"=w236, "Instrument.lvclass"=w237, "S4ACS_GUI in"=w300) -> ("error out"=w297:errorcluster, "S4ACS_GUI out"=w287:refnum<class "S4GUI.lvclass">)  [unwired: 7 in]
          n117 = Bundle By Name(cluster=w287, "Obs_state"=w284) -> (w286:refnum<class "S4GUI.lvclass">)
        }
        frame 202 {
          # "Dispara o comando para o dispositivo corrente."
          n118 = call "Read Instrument.lvclass.vi"("error in (no error)"=w320, "S4ACS_GUI in"=w321) -> ("error out"=w326:errorcluster, "Instrument.lvclass"=w327:refnum<class "Instrument.lvclass">, "S4ACS_GUI out"=w323:refnum<class "S4GUI.lvclass">)  [unwired: 7 in]
          n119 = call "Read CALW.vi"("error in (no error)"=w326, "Instrument in"=w327) -> ("error out"=w313:errorcluster, "Opt_Selector.lvclass"=w312:refnum<class "Opt_Selector.lvclass">, "Instrument out"=w325:refnum<class "Instrument.lvclass">)  [unwired: 7 in]
          n120 = call-dynamic "Read State Machine.vi"("error in (no error)"=w313, "Device in"=w312) -> ("error out"=w316:errorcluster, "State Machine.lvclass"=w318:refnum<class "State Machine.lvclass">, "Device out"=w310:refnum<class "Opt_Selector.lvclass">)  [unwired: 7 in]
          n121 = call "Next State.vi"("error in (no error)"=w316, "New_State"=1, "State Machine in"=w318) -> ("error out"=w315:errorcluster, "State Machine out"=w314:refnum<class "State Machine.lvclass">)  [unwired: 7 in]
          n122 = call-dynamic "Write State Machine.vi"("error in (no error)"=w315, "State Machine.lvclass"=w314, "Device in"=w310) -> ("error out"=w309:errorcluster, "Device out"=w311:refnum<class "Opt_Selector.lvclass">)  [unwired: 7 in]
          n123 = Increment(x=w307) -> (x+1=w306:u32)
          n124 = call "Write CALW.vi"("error in (no error)"=w309, "Opt_Selector.lvclass"=w311, "Instrument in"=w325) -> ("error out"=w322:errorcluster, "Instrument out"=w324:refnum<class "Instrument.lvclass">)  [unwired: 7 in]
          n125 = call "Write Instrument.lvclass.vi"("error in (no error)"=w322, "Instrument.lvclass"=w324, "S4ACS_GUI in"=w323) -> ("error out"=w319:errorcluster, "S4ACS_GUI out"=w308:refnum<class "S4GUI.lvclass">)  [unwired: 7 in]
          n126 = Bundle By Name(cluster=w308, "Obs_state"=w306) -> (w305:refnum<class "S4GUI.lvclass">)
        }
        frame 203 {
          # "Espera terminar a execução do comando atual \nantes de ir ao proximo passo da Observação."
          n127 = call "Read Instrument.lvclass.vi"("error in (no error)"=w346, "S4ACS_GUI in"=w347) -> ("error out"=w352:errorcluster, "Instrument.lvclass"=w353:refnum<class "Instrument.lvclass">, "S4ACS_GUI out"=w349:refnum<class "S4GUI.lvclass">)  [unwired: 7 in]
          n128 = call "Read CALW.vi"("error in (no error)"=w352, "Instrument in"=w353) -> ("error out"=w340:errorcluster, "Opt_Selector.lvclass"=w339:refnum<class "Opt_Selector.lvclass">, "Instrument out"=w351:refnum<class "Instrument.lvclass">)  [unwired: 7 in]
          n129 = call-dynamic "Read State Machine.vi"("error in (no error)"=w340, "Device in"=w339) -> ("error out"=w343:errorcluster, "State Machine.lvclass"=w344:refnum<class "State Machine.lvclass">, "Device out"=w337:refnum<class "Opt_Selector.lvclass">)  [unwired: 7 in]
          n130 = Increment(x=w330) -> (x+1=w329:u32)
          n131 = call-dynamic "Read State.vi"("error in (no error)"=w343, "State Machine in"=w344) -> ("error out"=w342:errorcluster, "State"=w332:i32, "State Machine out"=w341:refnum<class "State Machine.lvclass">)  [unwired: 7 in]
          n132 = Equal To 0?(x=w332) -> (x = 0?=w333:bool)
          n133 = call-dynamic "Write State Machine.vi"("error in (no error)"=w342, "State Machine.lvclass"=w341, "Device in"=w337) -> ("error out"=w336:errorcluster, "Device out"=w338:refnum<class "Opt_Selector.lvclass">)  [unwired: 7 in]
          n134 = call "Write CALW.vi"("error in (no error)"=w336, "Opt_Selector.lvclass"=w338, "Instrument in"=w351) -> ("error out"=w348:errorcluster, "Instrument out"=w350:refnum<class "Instrument.lvclass">)  [unwired: 7 in]
          n135 = Select(t=w329, s=w333, f=w330) -> (s? t:f=w331:u32)
          n136 = call "Write Instrument.lvclass.vi"("error in (no error)"=w348, "Instrument.lvclass"=w350, "S4ACS_GUI in"=w349) -> ("error out"=w345:errorcluster, "S4ACS_GUI out"=w335:refnum<class "S4GUI.lvclass">)  [unwired: 7 in]
          n137 = Bundle By Name(cluster=w335, "Obs_state"=w331) -> (w334:refnum<class "S4GUI.lvclass">)
        }
        frame 204 {
          # "Dispara o comando para o dispositivo corrente."
          n138 = call "Read Instrument.lvclass.vi"("error in (no error)"=w370, "S4ACS_GUI in"=w371) -> ("error out"=w376:errorcluster, "Instrument.lvclass"=w377:refnum<class "Instrument.lvclass">, "S4ACS_GUI out"=w373:refnum<class "S4GUI.lvclass">)  [unwired: 7 in]
          n139 = call "Read WPSEL.vi"("error in (no error)"=w376, "Instrument in"=w377) -> ("error out"=w363:errorcluster, "Opt_Selector.lvclass"=w362:refnum<class "Opt_Selector.lvclass">, "Instrument out"=w375:refnum<class "Instrument.lvclass">)  [unwired: 7 in]
          n140 = call-dynamic "Read State Machine.vi"("error in (no error)"=w363, "Device in"=w362) -> ("error out"=w366:errorcluster, "State Machine.lvclass"=w368:refnum<class "State Machine.lvclass">, "Device out"=w360:refnum<class "Opt_Selector.lvclass">)  [unwired: 7 in]
          n141 = call "Next State.vi"("error in (no error)"=w366, "New_State"=1, "State Machine in"=w368) -> ("error out"=w365:errorcluster, "State Machine out"=w364:refnum<class "State Machine.lvclass">)  [unwired: 7 in]
          n142 = call-dynamic "Write State Machine.vi"("error in (no error)"=w365, "State Machine.lvclass"=w364, "Device in"=w360) -> ("error out"=w359:errorcluster, "Device out"=w361:refnum<class "Opt_Selector.lvclass">)  [unwired: 7 in]
          n143 = Increment(x=w357) -> (x+1=w356:u32)
          n144 = call "Write WPSEL.vi"("error in (no error)"=w359, "Opt_Selector.lvclass"=w361, "Instrument in"=w375) -> ("error out"=w372:errorcluster, "Instrument out"=w374:refnum<class "Instrument.lvclass">)  [unwired: 7 in]
          n145 = call "Write Instrument.lvclass.vi"("error in (no error)"=w372, "Instrument.lvclass"=w374, "S4ACS_GUI in"=w373) -> ("error out"=w369:errorcluster, "S4ACS_GUI out"=w358:refnum<class "S4GUI.lvclass">)  [unwired: 7 in]
          n146 = Bundle By Name(cluster=w358, "Obs_state"=w356) -> (w355:refnum<class "S4GUI.lvclass">)
        }
        frame 205 {
          # "Espera terminar a execução do comando atual \nantes de ir ao proximo passo da Observação."
          n147 = call "Read Instrument.lvclass.vi"("error in (no error)"=w396, "S4ACS_GUI in"=w397) -> ("error out"=w402:errorcluster, "Instrument.lvclass"=w403:refnum<class "Instrument.lvclass">, "S4ACS_GUI out"=w399:refnum<class "S4GUI.lvclass">)  [unwired: 7 in]
          n148 = call "Read WPSEL.vi"("error in (no error)"=w402, "Instrument in"=w403) -> ("error out"=w390:errorcluster, "Opt_Selector.lvclass"=w389:refnum<class "Opt_Selector.lvclass">, "Instrument out"=w401:refnum<class "Instrument.lvclass">)  [unwired: 7 in]
          n149 = call-dynamic "Read State Machine.vi"("error in (no error)"=w390, "Device in"=w389) -> ("error out"=w393:errorcluster, "State Machine.lvclass"=w394:refnum<class "State Machine.lvclass">, "Device out"=w387:refnum<class "Opt_Selector.lvclass">)  [unwired: 7 in]
          n150 = Increment(x=w380) -> (x+1=w379:u32)
          n151 = call-dynamic "Read State.vi"("error in (no error)"=w393, "State Machine in"=w394) -> ("error out"=w392:errorcluster, "State"=w382:i32, "State Machine out"=w391:refnum<class "State Machine.lvclass">)  [unwired: 7 in]
          n152 = Equal To 0?(x=w382) -> (x = 0?=w383:bool)
          n153 = call-dynamic "Write State Machine.vi"("error in (no error)"=w392, "State Machine.lvclass"=w391, "Device in"=w387) -> ("error out"=w386:errorcluster, "Device out"=w388:refnum<class "Opt_Selector.lvclass">)  [unwired: 7 in]
          n154 = call "Write WPSEL.vi"("error in (no error)"=w386, "Opt_Selector.lvclass"=w388, "Instrument in"=w401) -> ("error out"=w398:errorcluster, "Instrument out"=w400:refnum<class "Instrument.lvclass">)  [unwired: 7 in]
          n155 = Select(t=w379, s=w383, f=w380) -> (s? t:f=w381:u32)
          n156 = call "Write Instrument.lvclass.vi"("error in (no error)"=w398, "Instrument.lvclass"=w400, "S4ACS_GUI in"=w399) -> ("error out"=w395:errorcluster, "S4ACS_GUI out"=w385:refnum<class "S4GUI.lvclass">)  [unwired: 7 in]
          n157 = Bundle By Name(cluster=w385, "Obs_state"=w381) -> (w384:refnum<class "S4GUI.lvclass">)
        }
        frame 206 {
          # "Dispara o comando para o dispositivo corrente."
          n158 = call "Read Instrument.lvclass.vi"("error in (no error)"=w419, "S4ACS_GUI in"=w420) -> ("error out"=w425:errorcluster, "Instrument.lvclass"=w426:refnum<class "Instrument.lvclass">, "S4ACS_GUI out"=w422:refnum<class "S4GUI.lvclass">)  [unwired: 7 in]
          n159 = call "Read WPSEL.vi"("error in (no error)"=w425, "Instrument in"=w426) -> ("error out"=w413:errorcluster, "Opt_Selector.lvclass"=w414:refnum<class "Opt_Selector.lvclass">, "Instrument out"=w424:refnum<class "Instrument.lvclass">)  [unwired: 7 in]
          n160 = call "Read target name.vi"("error in (no error)"=w413, "Optics in"=w414) -> ("error out"=w407:errorcluster, "target name"=w412:string, "Optics out"=w406:refnum<class "Opt_Selector.lvclass">)  [unwired: 7 in]
          n161 = Equal?(x=w412, y="OFF") -> (x = y?=w410:bool)
          n162 = Increment(x=w416) -> (x+1=w408:u32)
          n163 = call "Write WPSEL.vi"("error in (no error)"=w407, "Opt_Selector.lvclass"=w406, "Instrument in"=w424) -> ("error out"=w421:errorcluster, "Instrument out"=w423:refnum<class "Instrument.lvclass">)  [unwired: 7 in]
          n164 = Select(t=u32 0, s=w410, f=w408) -> (s? t:f=w405:u32)
          n165 = call "Write Instrument.lvclass.vi"("error in (no error)"=w421, "Instrument.lvclass"=w423, "S4ACS_GUI in"=w422) -> ("error out"=w418:errorcluster, "S4ACS_GUI out"=w417:refnum<class "S4GUI.lvclass">)  [unwired: 7 in]
          n166 = Bundle By Name(cluster=w417, "Obs_state"=w405) -> (w415:refnum<class "S4GUI.lvclass">)
        }
        frame 207 {
          # "Dispara o comando para o dispositivo corrente."
          n167 = call "Read Instrument.lvclass.vi"("error in (no error)"=w443, "S4ACS_GUI in"=w444) -> ("error out"=w449:errorcluster, "Instrument.lvclass"=w450:refnum<class "Instrument.lvclass">, "S4ACS_GUI out"=w446:refnum<class "S4GUI.lvclass">)  [unwired: 7 in]
          n168 = call "Read WPROT.vi"("error in (no error)"=w449, "Instrument in"=w450) -> ("error out"=w436:errorcluster, "Opt_Selector.lvclass"=w435:refnum<class "Opt_Selector.lvclass">, "Instrument out"=w448:refnum<class "Instrument.lvclass">)  [unwired: 7 in]
          n169 = call-dynamic "Read State Machine.vi"("error in (no error)"=w436, "Device in"=w435) -> ("error out"=w439:errorcluster, "State Machine.lvclass"=w441:refnum<class "State Machine.lvclass">, "Device out"=w433:refnum<class "Opt_Selector.lvclass">)  [unwired: 7 in]
          n170 = call "Next State.vi"("error in (no error)"=w439, "New_State"=1, "State Machine in"=w441) -> ("error out"=w438:errorcluster, "State Machine out"=w437:refnum<class "State Machine.lvclass">)  [unwired: 7 in]
          n171 = call-dynamic "Write State Machine.vi"("error in (no error)"=w438, "State Machine.lvclass"=w437, "Device in"=w433) -> ("error out"=w432:errorcluster, "Device out"=w434:refnum<class "Opt_Selector.lvclass">)  [unwired: 7 in]
          n172 = Increment(x=w430) -> (x+1=w429:u32)
          n173 = call "Write WPROT.vi"("error in (no error)"=w432, "Opt_Selector.lvclass"=w434, "Instrument in"=w448) -> ("error out"=w445:errorcluster, "Instrument out"=w447:refnum<class "Instrument.lvclass">)  [unwired: 7 in]
          n174 = call "Write Instrument.lvclass.vi"("error in (no error)"=w445, "Instrument.lvclass"=w447, "S4ACS_GUI in"=w446) -> ("error out"=w442:errorcluster, "S4ACS_GUI out"=w431:refnum<class "S4GUI.lvclass">)  [unwired: 7 in]
          n175 = Bundle By Name(cluster=w431, "Obs_state"=w429) -> (w428:refnum<class "S4GUI.lvclass">)
        }
        frame 208 {
          # "Espera terminar a execução do comando atual \nantes de ir ao proximo passo da Observação."
          n176 = call "Read Instrument.lvclass.vi"("error in (no error)"=w469, "S4ACS_GUI in"=w470) -> ("error out"=w475:errorcluster, "Instrument.lvclass"=w476:refnum<class "Instrument.lvclass">, "S4ACS_GUI out"=w472:refnum<class "S4GUI.lvclass">)  [unwired: 7 in]
          n177 = call "Read WPROT.vi"("error in (no error)"=w475, "Instrument in"=w476) -> ("error out"=w463:errorcluster, "Opt_Selector.lvclass"=w462:refnum<class "Opt_Selector.lvclass">, "Instrument out"=w474:refnum<class "Instrument.lvclass">)  [unwired: 7 in]
          n178 = call-dynamic "Read State Machine.vi"("error in (no error)"=w463, "Device in"=w462) -> ("error out"=w466:errorcluster, "State Machine.lvclass"=w467:refnum<class "State Machine.lvclass">, "Device out"=w460:refnum<class "Opt_Selector.lvclass">)  [unwired: 7 in]
          n179 = call-dynamic "Read State.vi"("error in (no error)"=w466, "State Machine in"=w467) -> ("error out"=w465:errorcluster, "State"=w455:i32, "State Machine out"=w464:refnum<class "State Machine.lvclass">)  [unwired: 7 in]
          n180 = Equal To 0?(x=w455) -> (x = 0?=w456:bool)
          n181 = call-dynamic "Write State Machine.vi"("error in (no error)"=w465, "State Machine.lvclass"=w464, "Device in"=w460) -> ("error out"=w459:errorcluster, "Device out"=w461:refnum<class "Opt_Selector.lvclass">)  [unwired: 7 in]
          n182 = call "Write WPSEL.vi"("error in (no error)"=w459, "Opt_Selector.lvclass"=w461, "Instrument in"=w474) -> ("error out"=w471:errorcluster, "Instrument out"=w473:refnum<class "Instrument.lvclass">)  [unwired: 7 in]
          n183 = Select(t=u32 0, s=w456, f=w453) -> (s? t:f=w454:u32)
          n184 = call "Write Instrument.lvclass.vi"("error in (no error)"=w471, "Instrument.lvclass"=w473, "S4ACS_GUI in"=w472) -> ("error out"=w468:errorcluster, "S4ACS_GUI out"=w458:refnum<class "S4GUI.lvclass">)  [unwired: 7 in]
          n185 = Bundle By Name(cluster=w458, "Obs_state"=w454) -> (w457:refnum<class "S4GUI.lvclass">)
        }
        frame 291 {
          # "configura o canal,\nmas não dispara\na exposicao."
          # "Dispara o comando para o dispositivo corrente."
          n186 = call-dynamic "Read Channel.vi"("error in (no error)"=w483, "Acquisition in"=w484) -> ("error out"=w489:errorcluster, "Channel.lvclass"=w491:refnum<class "Channel.lvclass">, "Acquisition out"=w499:refnum<class "Acquisition.lvclass">)  [unwired: 7 in]
          n187 = call-dynamic "Write expose.vi"("error in (no error)"=w489, "expose"=FALSE, "Channel in"=w491) -> ("error out"=w488:errorcluster, "Channel out"=w490:refnum<class "Channel.lvclass">)  [unwired: 7 in]
          n188 = call-dynamic "Read State Machine.vi"("error in (no error)"=w488, "Device in"=w490) -> ("error out"=w496:errorcluster, "State Machine.lvclass"=w498:refnum<class "State Machine.lvclass">, "Device out"=w494:refnum<class "Channel.lvclass">)  [unwired: 7 in]
          n189 = call "Next State.vi"("error in (no error)"=w496, "New_State"=1, "State Machine in"=w498) -> ("error out"=w485:errorcluster, "State Machine out"=w486:refnum<class "State Machine.lvclass">)  [unwired: 7 in]
          n190 = call-dynamic "Write State Machine.vi"("error in (no error)"=w485, "State Machine.lvclass"=w486, "Device in"=w494) -> ("error out"=w493:errorcluster, "Device out"=w495:refnum<class "Channel.lvclass">)  [unwired: 7 in]
          n191 = call-dynamic "Write Channel.vi"("error in (no error)"=w493, "Channel.lvclass"=w495, "Acquisition in"=w499) -> ("error out"=w478:errorcluster, "Acquisition out"=w481:refnum<class "Acquisition.lvclass">)  [unwired: 7 in]
          n192 = Increment(x=w492) -> (x+1=w482:u32)
          n193 = call-dynamic "Write Acq_state.vi"("error in (no error)"=w478, "Acq_state"=w482, "Acquisition in"=w481) -> ("error out"=w477:errorcluster, "Acquisition out"=w480:refnum<class "Acquisition.lvclass">)  [unwired: 7 in]
        }
        frame 292 {
          # "Espera terminar a execução do comando atual \nantes de ir ao proximo passo da Observação."
          n194 = call-dynamic "Read Channel.vi"("error in (no error)"=w500, "Acquisition in"=w507) -> ("error out"=w520:errorcluster, "Channel.lvclass"=w519:refnum<class "Channel.lvclass">, "Acquisition out"=w521:refnum<class "Acquisition.lvclass">)  [unwired: 7 in]
          n195 = call-dynamic "Read State Machine.vi"("error in (no error)"=w520, "Device in"=w519) -> ("error out"=w513:errorcluster, "State Machine.lvclass"=w515:refnum<class "State Machine.lvclass">, "Device out"=w517:refnum<class "Channel.lvclass">)  [unwired: 7 in]
          n196 = call-dynamic "Read State.vi"("error in (no error)"=w513, "State Machine in"=w515) -> ("error out"=w512:errorcluster, "State"=w510:i32, "State Machine out"=w514:refnum<class "State Machine.lvclass">)  [unwired: 7 in]
          n197 = Equal To 0?(x=w510) -> (x = 0?=w511:bool)
          n198 = call-dynamic "Write State Machine.vi"("error in (no error)"=w512, "State Machine.lvclass"=w514, "Device in"=w517) -> ("error out"=w516:errorcluster, "Device out"=w518:refnum<class "Channel.lvclass">)  [unwired: 7 in]
          n199 = call-dynamic "Write Channel.vi"("error in (no error)"=w516, "Channel.lvclass"=w518, "Acquisition in"=w521) -> ("error out"=w504:errorcluster, "Acquisition out"=w503:refnum<class "Acquisition.lvclass">)  [unwired: 7 in]
          n200 = Select(t=u32 299, s=w511, f=w508) -> (s? t:f=w505:u32)
          n201 = call-dynamic "Write Acq_state.vi"("error in (no error)"=w504, "Acq_state"=w505, "Acquisition in"=w503) -> ("error out"=w501:errorcluster, "Acquisition out"=w502:refnum<class "Acquisition.lvclass">)  [unwired: 7 in]
        }
        frame 299 {
          # "Verifica se é modo fotometria ou polarimetria:\nTrue = polarimetria\nFalse = fotometria"
          n202 = call "Read Instrument.lvclass.vi"("error in (no error)"=w533, "S4ACS_GUI in"=w534) -> ("error out"=w530:errorcluster, "Instrument.lvclass"=w531:refnum<class "Instrument.lvclass">, "S4ACS_GUI out"=w527:refnum<class "S4GUI.lvclass">)  [unwired: 7 in]
          n203 = call-dynamic "Read mode.vi"("error in (no error)"=w530, "Instrument in"=w531) -> ("error out"=w525:errorcluster, "mode"=w529:bool)  [unwired: 7 in, 1 out]
          n204 = Select(t=u32 301, s=w529, f=u32 321 ("t")) -> (s? t:f=w526:u32)
          n205 = call-dynamic "Write Acq_state.vi"("error in (no error)"=w525, "Acq_state"=w526, "Acquisition in"=w524) -> ("error out"=w523:errorcluster, "Acquisition out"=w522:refnum<class "Acquisition.lvclass">)  [unwired: 7 in]
        }
        frame 301 {
          n206 = call "Read Instrument.lvclass.vi"("error in (no error)"=w571, "S4ACS_GUI in"=w572) -> ("error out"=w575:errorcluster, "Instrument.lvclass"=w576:refnum<class "Instrument.lvclass">, "S4ACS_GUI out"=w573:refnum<class "S4GUI.lvclass">)  [unwired: 7 in]
          n207 = call "Read WPROT.vi"("error in (no error)"=w575, "Instrument in"=w576) -> ("error out"=w568:errorcluster, "Opt_Selector.lvclass"=w569:refnum<class "Opt_Selector.lvclass">, "Instrument out"=w574:refnum<class "Instrument.lvclass">)  [unwired: 7 in]
          n208 = call-dynamic "getTargetPos.vi"("error in (no error)"=w568, "Opt_Selector in"=w569) -> ("error out"=w567:errorcluster, "Target Pos"=w547:u16, "Opt_Selector out"=w566:refnum<class "Opt_Selector.lvclass">)  [unwired: 7 in]
          n209 = Build Array(-1.0 ("element"), 0.0 ("element"), 22.5 ("element"), 45.0 ("element"), 67.5 ("element"), 90.0 ("element"), 112.5 ("element"), 135.0 ("element"), 157.5 ("element"), 180.0 ("element"), 202.5 ("element"), 225.0 ("element"), 247.5 ("element"), 270.0 ("element"), 292.5 ("element"), 315.0 ("element"), 337.5 ("element")) -> (w559:dbl[])
          n210 = Index Array(array=w559, index=w547) -> (element=w546:dbl)
          n211 = case shown="1..16" w547 {
            selector: w547 -> [_ w599]
            tunnel: w574 -> [w584 w587]
            tunnel: [w584 w587] -> w542
            tunnel: [w581 w586] -> w541
            tunnel: w570 -> [_ w601]
            tunnel: [u32 311 w600] -> w540
            tunnel: w567 -> [w582 w595]
            tunnel: w566 -> [w583 w594]
            tunnel: w546 -> [_ w589]
            tunnel: [w579 w588] -> w543
            frame 0, Default {
              # "Verifica os ciclos"
              # "Recupera a sequencia anterior para o caso \nde repetição da sequencia (sem precisar clicar \nnas posicoes desejadas novamente)."
              n212 = call-dynamic "Read sequencia_ant.vi"("error in (no error)"=w582, "Opt_Selector in"=w583) -> ("error out"=w578:errorcluster, "sequencia_ant"=w577:u16, "Opt_Selector out"=w580:refnum<class "Opt_Selector.lvclass">)  [unwired: 7 in]
              n213 = call-dynamic "Write sequencia.vi"("error in (no error)"=w578, "sequencia"=w577, "Opt_Selector in"=w580) -> ("error out"=w581:errorcluster, "Opt_Selector out"=w579:refnum<class "Opt_Selector.lvclass">)  [unwired: 7 in]
            }
            frame 1..16 {
              n214 = Number To Decimal String(number=w599) -> (decimal integer string=w598:string)  [unwired: 1 in]
              n215 = Concatenate Strings("WP" ("string"), w598) -> (w596:string)
              n216 = call "Write target name.vi"("error in (no error)"=w595, "target name"=w596, "Optics in"=w594) -> ("error out"=w592:errorcluster, "Optics out"=w593:refnum<class "Opt_Selector.lvclass">)  [unwired: 7 in]
              n217 = call "Write target.vi"("error in (no error)"=w592, "target"=w589, "Optics in"=w593) -> ("error out"=w591:errorcluster, "Optics out"=w590:refnum<class "Opt_Selector.lvclass">)  [unwired: 7 in]
              n218 = call-dynamic "Read State Machine.vi"("error in (no error)"=w591, "Device in"=w590) -> ("error out"=w605:errorcluster, "State Machine.lvclass"=w607:refnum<class "State Machine.lvclass">, "Device out"=w602:refnum<class "Opt_Selector.lvclass">)  [unwired: 7 in]
              n219 = Increment(x=w601) -> (x+1=w600:u32)
              n220 = call "Next State.vi"("error in (no error)"=w605, "New_State"=1, "State Machine in"=w607) -> ("error out"=w604:errorcluster, "State Machine out"=w603:refnum<class "State Machine.lvclass">)  [unwired: 7 in]
              n221 = call-dynamic "Write State Machine.vi"("error in (no error)"=w604, "State Machine.lvclass"=w603, "Device in"=w602) -> ("error out"=w586:errorcluster, "Device out"=w588:refnum<class "Opt_Selector.lvclass">)  [unwired: 7 in]
            }
          }
          n222 = call "Write WPROT.vi"("error in (no error)"=w541, "Opt_Selector.lvclass"=w543, "Instrument in"=w542) -> ("error out"=w545:errorcluster, "Instrument out"=w544:refnum<class "Instrument.lvclass">)  [unwired: 7 in]
          n223 = call "Write Instrument.lvclass.vi"("error in (no error)"=w545, "Instrument.lvclass"=w544, "S4ACS_GUI in"=w573) -> ("error out"=w538:errorcluster, "S4ACS_GUI out"=w537:refnum<class "S4GUI.lvclass">)  [unwired: 7 in]
          n224 = call-dynamic "Write Acq_state.vi"("error in (no error)"=w538, "Acq_state"=w540, "Acquisition in"=w539) -> ("error out"=w536:errorcluster, "Acquisition out"=w535:refnum<class "Acquisition.lvclass">)  [unwired: 7 in]
        }
        frame 302 {
          # "TESTE: 1 x 20ms = 0.02s de pausa entre \nposições do waveplate."
          # "Espera terminar o movimento para a posição \"target\" do waveplate\nantes de ir para o estado de pausa."
          n225 = call "Read Instrument.lvclass.vi"("error in (no error)"=w630, "S4ACS_GUI in"=w631) -> ("error out"=w636:errorcluster, "Instrument.lvclass"=w637:refnum<class "Instrument.lvclass">, "S4ACS_GUI out"=w633:refnum<class "S4GUI.lvclass">)  [unwired: 7 in]
          n226 = call "Read WPROT.vi"("error in (no error)"=w636, "Instrument in"=w637) -> ("error out"=w627:errorcluster, "Opt_Selector.lvclass"=w626:refnum<class "Opt_Selector.lvclass">, "Instrument out"=w635:refnum<class "Instrument.lvclass">)  [unwired: 7 in]
          n227 = call-dynamic "Read State Machine.vi"("error in (no error)"=w627, "Device in"=w626) -> ("error out"=w628:errorcluster, "State Machine.lvclass"=w629:refnum<class "State Machine.lvclass">, "Device out"=w624:refnum<class "Opt_Selector.lvclass">)  [unwired: 7 in]
          n228 = Increment(x=w620) -> (x+1=w619:u32)
          n229 = call-dynamic "Read State.vi"("error in (no error)"=w628, "State Machine in"=w629) -> ("error out"=w614:errorcluster, "State"=w621:i32, "State Machine out"=w618:refnum<class "State Machine.lvclass">)  [unwired: 7 in]
          n230 = Equal To 0?(x=w621) -> (x = 0?=w622:bool)
          n231 = call-dynamic "Write Timer.vi"("error in (no error)"=w614, "Timer"=u32 1, "State Machine in"=w618) -> ("error out"=w615:errorcluster, "State Machine out"=w617:refnum<class "State Machine.lvclass">)  [unwired: 7 in]
          n232 = call-dynamic "Write State Machine.vi"("error in (no error)"=w615, "State Machine.lvclass"=w617, "Device in"=w624) -> ("error out"=w623:errorcluster, "Device out"=w625:refnum<class "Opt_Selector.lvclass">)  [unwired: 7 in]
          n233 = call "Write WPROT.vi"("error in (no error)"=w623, "Opt_Selector.lvclass"=w625, "Instrument in"=w635) -> ("error out"=w632:errorcluster, "Instrument out"=w634:refnum<class "Instrument.lvclass">)  [unwired: 7 in]
          n234 = Select(t=w619, s=w622, f=w620) -> (s? t:f=w613:u32)
          n235 = call "Write Instrument.lvclass.vi"("error in (no error)"=w632, "Instrument.lvclass"=w634, "S4ACS_GUI in"=w633) -> ("error out"=w611:errorcluster, "S4ACS_GUI out"=w608:refnum<class "S4GUI.lvclass">)  [unwired: 7 in]
          n236 = call-dynamic "Write Acq_state.vi"("error in (no error)"=w611, "Acq_state"=w613, "Acquisition in"=w612) -> ("error out"=w610:errorcluster, "Acquisition out"=w609:refnum<class "Acquisition.lvclass">)  [unwired: 7 in]
        }
        frame 303 {
          # "Espera terminar a pausa carregada no Timer"
          n237 = call "Read Instrument.lvclass.vi"("error in (no error)"=w656, "S4ACS_GUI in"=w657) -> ("error out"=w662:errorcluster, "Instrument.lvclass"=w663:refnum<class "Instrument.lvclass">, "S4ACS_GUI out"=w659:refnum<class "S4GUI.lvclass">)  [unwired: 7 in]
          n238 = call "Read WPROT.vi"("error in (no error)"=w662, "Instrument in"=w663) -> ("error out"=w655:errorcluster, "Opt_Selector.lvclass"=w654:refnum<class "Opt_Selector.lvclass">, "Instrument out"=w661:refnum<class "Instrument.lvclass">)  [unwired: 7 in]
          n239 = call-dynamic "Read State Machine.vi"("error in (no error)"=w655, "Device in"=w654) -> ("error out"=w647:errorcluster, "State Machine.lvclass"=w648:refnum<class "State Machine.lvclass">, "Device out"=w652:refnum<class "Opt_Selector.lvclass">)  [unwired: 7 in]
          n240 = Increment(x=w644) -> (x+1=w649:u32)
          n241 = call "Verify Timer.vi"("error in (no error)"=w647, "State Machine in"=w648) -> ("error out"=w645:errorcluster, "timeout"=w650:bool, "State Machine out"=w646:refnum<class "State Machine.lvclass">)  [unwired: 7 in]
          n242 = call-dynamic "Write State Machine.vi"("error in (no error)"=w645, "State Machine.lvclass"=w646, "Device in"=w652) -> ("error out"=w651:errorcluster, "Device out"=w653:refnum<class "Opt_Selector.lvclass">)  [unwired: 7 in]
          n243 = call "Write WPROT.vi"("error in (no error)"=w651, "Opt_Selector.lvclass"=w653, "Instrument in"=w661) -> ("error out"=w658:errorcluster, "Instrument out"=w660:refnum<class "Instrument.lvclass">)  [unwired: 7 in]
          n244 = call "Write Instrument.lvclass.vi"("error in (no error)"=w658, "Instrument.lvclass"=w660, "S4ACS_GUI in"=w659) -> ("error out"=w642:errorcluster, "S4ACS_GUI out"=w643:refnum<class "S4GUI.lvclass">)  [unwired: 7 in]
          n245 = Select(t=w649, s=w650, f=w644) -> (s? t:f=w641:u32)
          n246 = call-dynamic "Write Acq_state.vi"("error in (no error)"=w642, "Acq_state"=w641, "Acquisition in"=w638) -> ("error out"=w639:errorcluster, "Acquisition out"=w640:refnum<class "Acquisition.lvclass">)  [unwired: 7 in]
        }
        frame 304 {
          n247 = call-dynamic "Read Sync Box.lvclass.vi"("error in (no error)"=w676, "SPARC4_AC in"=w677) -> ("error out"=w666:errorcluster, "Sync Box.lvclass"=w668:refnum<class "Sync Box.lvclass">, "SPARC4_AC out"=w679:refnum<class "S4GUI.lvclass">)  [unwired: 7 in]
          n248 = call "Read connection.vi"("error in (no error)"=w666, "Server in"=w668) -> ("error out"=w665:errorcluster, "connection"=w664:bool, "Server out"=w667:refnum<class "Sync Box.lvclass">)  [unwired: 7 in]
          n249 = case shown="True" w664 {
            tunnel: [w685 w694] -> w680
            tunnel: [w684 w693] -> w678
            tunnel: w675 -> [w683 w692]
            tunnel: [w681 w691] -> w673
            tunnel: w667 -> [w685 w687]
            tunnel: w665 -> [w684 w686]
            frame False {
              # "SyncBox not connected: skip SyncBox configuration"
              n250 = Increment(x=w683) -> (x+1=w682:u32)
              n251 = Increment(x=w682) -> (x+1=w681:u32)
            }
            frame True {
              # "SyncBox connected: performs SyncBox configuration"
              # "SyncBox ocupado?"
              n252 = call-dynamic "Read busy.vi"("error in (no error)"=w686, "Sync Box in"=w687) -> ("error out"=w688:errorcluster, "busy"=w690:bool, "Sync Box out"=w689:refnum<class "Sync Box.lvclass">)  [unwired: 7 in]
              n253 = case shown="False" w690 {
                tunnel: w688 -> [w717 w718]
                tunnel: [w698 w719] -> w694
                tunnel: [w696 w718] -> w693
                tunnel: w692 -> [w707 w720]
                tunnel: w689 -> [w701 w719]
                tunnel: [w700 w720] -> w691
                frame False {
                  # "configura delays do syncBox"
                  # "Dispara o comando para o dispositivo corrente."
                  n254 = call-dynamic "Read Trigger.lvclass.vi"("error in (no error)"=w717, "Sync Box in"=w701) -> ("error out"=w712:errorcluster, "Trigger.lvclass"=w711:refnum<class "Trigger.lvclass">, "Sync Box out"=w716:refnum<class "Sync Box.lvclass">)  [unwired: 7 in]
                  n255 = call-dynamic "Read State Machine.vi"("error in (no error)"=w712, "Device in"=w711) -> ("error out"=w713:errorcluster, "State Machine.lvclass"=w715:refnum<class "State Machine.lvclass">, "Device out"=w709:refnum<class "Trigger.lvclass">)  [unwired: 7 in]
                  n256 = call "Next State.vi"("error in (no error)"=w713, "New_State"=10, "State Machine in"=w715) -> ("error out"=w703:errorcluster, "State Machine out"=w705:refnum<class "State Machine.lvclass">)  [unwired: 7 in]
                  n257 = call-dynamic "Write Timer.vi"("error in (no error)"=w703, "Timer"=u32 5, "State Machine in"=w705) -> ("error out"=w702:errorcluster, "State Machine out"=w704:refnum<class "State Machine.lvclass">)  [unwired: 7 in]
                  n258 = call-dynamic "Write State Machine.vi"("error in (no error)"=w702, "State Machine.lvclass"=w704, "Device in"=w709) -> ("error out"=w708:errorcluster, "Device out"=w710:refnum<class "Trigger.lvclass">)  [unwired: 7 in]
                  n259 = Increment(x=w707) -> (x+1=w700:u32)
                  n260 = call-dynamic "Write Trigger.lvclass.vi"("error in (no error)"=w708, "Trigger.lvclass"=w710, "Sync Box in"=w716) -> ("error out"=w697:errorcluster, "Sync Box out"=w699:refnum<class "Sync Box.lvclass">)  [unwired: 7 in]
                  n261 = call-dynamic "Write busy.vi"("error in (no error)"=w697, "busy"=TRUE, "Sync Box in"=w699) -> ("error out"=w696:errorcluster, "Sync Box out"=w698:refnum<class "Sync Box.lvclass">)  [unwired: 7 in]
                }
                frame True {
                }
              }
            }
          }
          n262 = call-dynamic "Write Sync Box.lvclass.vi"("error in (no error)"=w678, "Sync Box.lvclass"=w680, "SPARC4_AC in"=w679) -> ("error out"=w672:errorcluster, "SPARC4_AC out"=w674:refnum<class "S4GUI.lvclass">)  [unwired: 7 in]
          n263 = call-dynamic "Write Acq_state.vi"("error in (no error)"=w672, "Acq_state"=w673, "Acquisition in"=w669) -> ("error out"=w670:errorcluster, "Acquisition out"=w671:refnum<class "Acquisition.lvclass">)  [unwired: 7 in]
        }
        frame 305 {
          # "Espera terminar a execução do comando atual \nantes de ir ao proximo passo da Observação."
          n264 = call-dynamic "Read Sync Box.lvclass.vi"("error in (no error)"=w743, "SPARC4_AC in"=w744) -> ("error out"=w747:errorcluster, "Sync Box.lvclass"=w748:refnum<class "Sync Box.lvclass">, "SPARC4_AC out"=w745:refnum<class "S4GUI.lvclass">)  [unwired: 7 in]
          n265 = call-dynamic "Read Trigger.lvclass.vi"("error in (no error)"=w747, "Sync Box in"=w748) -> ("error out"=w742:errorcluster, "Trigger.lvclass"=w741:refnum<class "Trigger.lvclass">, "Sync Box out"=w746:refnum<class "Sync Box.lvclass">)  [unwired: 7 in]
          n266 = call-dynamic "Read State Machine.vi"("error in (no error)"=w742, "Device in"=w741) -> ("error out"=w735:errorcluster, "State Machine.lvclass"=w737:refnum<class "State Machine.lvclass">, "Device out"=w739:refnum<class "Trigger.lvclass">)  [unwired: 7 in]
          n267 = call-dynamic "Read State.vi"("error in (no error)"=w735, "State Machine in"=w737) -> ("error out"=w734:errorcluster, "State"=w733:i32, "State Machine out"=w736:refnum<class "State Machine.lvclass">)  [unwired: 7 in]
          n268 = Equal To 0?(x=w733) -> (x = 0?=w731:bool)
          n269 = call-dynamic "Write State Machine.vi"("error in (no error)"=w734, "State Machine.lvclass"=w736, "Device in"=w739) -> ("error out"=w738:errorcluster, "Device out"=w740:refnum<class "Trigger.lvclass">)  [unwired: 7 in]
          n270 = call-dynamic "Write Trigger.lvclass.vi"("error in (no error)"=w738, "Trigger.lvclass"=w740, "Sync Box in"=w746) -> ("error out"=w729:errorcluster, "Sync Box out"=w730:refnum<class "Sync Box.lvclass">)  [unwired: 7 in]
          n271 = case shown="True" w731 {
            tunnel: [w751 w757] -> w725
            tunnel: w732 -> [w751 w758]
            tunnel: w730 -> [w750 w756]
            tunnel: w729 -> [w749 w755]
            tunnel: [w749 w754] -> w728
            tunnel: [w750 w753] -> w727
            frame False {
            }
            frame True {
              # "Sinaliza que SyncBox\nficou livre."
              n272 = Increment(x=w758) -> (x+1=w757:u32)
              n273 = call-dynamic "Write busy.vi"("error in (no error)"=w755, "busy"=FALSE, "Sync Box in"=w756) -> ("error out"=w754:errorcluster, "Sync Box out"=w753:refnum<class "Sync Box.lvclass">)  [unwired: 7 in]
            }
          }
          n274 = call-dynamic "Write Sync Box.lvclass.vi"("error in (no error)"=w728, "Sync Box.lvclass"=w727, "SPARC4_AC in"=w745) -> ("error out"=w724:errorcluster, "SPARC4_AC out"=w726:refnum<class "S4GUI.lvclass">)  [unwired: 7 in]
          n275 = call-dynamic "Write Acq_state.vi"("error in (no error)"=w724, "Acq_state"=w725, "Acquisition in"=w723) -> ("error out"=w721:errorcluster, "Acquisition out"=w722:refnum<class "Acquisition.lvclass">)  [unwired: 7 in]
        }
        frame 306 {
          # "Dispara o comando para o dispositivo corrente."
          n276 = call-dynamic "Read Channel.vi"("error in (no error)"=w765, "Acquisition in"=w766) -> ("error out"=w777:errorcluster, "Channel.lvclass"=w776:refnum<class "Channel.lvclass">, "Acquisition out"=w781:refnum<class "Acquisition.lvclass">)  [unwired: 7 in]
          n277 = call-dynamic "Read State Machine.vi"("error in (no error)"=w777, "Device in"=w776) -> ("error out"=w778:errorcluster, "State Machine.lvclass"=w780:refnum<class "State Machine.lvclass">, "Device out"=w774:refnum<class "Channel.lvclass">)  [unwired: 7 in]
          n278 = call "Next State.vi"("error in (no error)"=w778, "New_State"=50, "State Machine in"=w780) -> ("error out"=w768:errorcluster, "State Machine out"=w770:refnum<class "State Machine.lvclass">)  [unwired: 7 in]
          n279 = call-dynamic "Write Timer.vi"("error in (no error)"=w768, "Timer"=u32 2, "State Machine in"=w770) -> ("error out"=w767:errorcluster, "State Machine out"=w769:refnum<class "State Machine.lvclass">)  [unwired: 7 in]
          n280 = call-dynamic "Write State Machine.vi"("error in (no error)"=w767, "State Machine.lvclass"=w769, "Device in"=w774) -> ("error out"=w773:errorcluster, "Device out"=w775:refnum<class "Channel.lvclass">)  [unwired: 7 in]
          n281 = Increment(x=w772) -> (x+1=w764:u32)
          n282 = call-dynamic "Write Channel.vi"("error in (no error)"=w773, "Channel.lvclass"=w775, "Acquisition in"=w781) -> ("error out"=w762:errorcluster, "Acquisition out"=w761:refnum<class "Acquisition.lvclass">)  [unwired: 7 in]
          n283 = call-dynamic "Write Acq_state.vi"("error in (no error)"=w762, "Acq_state"=w764, "Acquisition in"=w761) -> ("error out"=w759:errorcluster, "Acquisition out"=w760:refnum<class "Acquisition.lvclass">)  [unwired: 7 in]
        }
        frame 307 {
          # "Espera terminar a pausa carregada no Timer"
          n284 = call "Read Instrument.lvclass.vi"("error in (no error)"=w800, "S4ACS_GUI in"=w801) -> ("error out"=w806:errorcluster, "Instrument.lvclass"=w807:refnum<class "Instrument.lvclass">, "S4ACS_GUI out"=w803:refnum<class "S4GUI.lvclass">)  [unwired: 7 in]
          n285 = call "Read WPROT.vi"("error in (no error)"=w806, "Instrument in"=w807) -> ("error out"=w799:errorcluster, "Opt_Selector.lvclass"=w798:refnum<class "Opt_Selector.lvclass">, "Instrument out"=w805:refnum<class "Instrument.lvclass">)  [unwired: 7 in]
          n286 = call-dynamic "Read State Machine.vi"("error in (no error)"=w799, "Device in"=w798) -> ("error out"=w791:errorcluster, "State Machine.lvclass"=w792:refnum<class "State Machine.lvclass">, "Device out"=w796:refnum<class "Opt_Selector.lvclass">)  [unwired: 7 in]
          n287 = Increment(x=w788) -> (x+1=w793:u32)
          n288 = call "Verify Timer.vi"("error in (no error)"=w791, "State Machine in"=w792) -> ("error out"=w789:errorcluster, "timeout"=w794:bool, "State Machine out"=w790:refnum<class "State Machine.lvclass">)  [unwired: 7 in]
          n289 = call-dynamic "Write State Machine.vi"("error in (no error)"=w789, "State Machine.lvclass"=w790, "Device in"=w796) -> ("error out"=w795:errorcluster, "Device out"=w797:refnum<class "Opt_Selector.lvclass">)  [unwired: 7 in]
          n290 = call "Write WPROT.vi"("error in (no error)"=w795, "Opt_Selector.lvclass"=w797, "Instrument in"=w805) -> ("error out"=w802:errorcluster, "Instrument out"=w804:refnum<class "Instrument.lvclass">)  [unwired: 7 in]
          n291 = call "Write Instrument.lvclass.vi"("error in (no error)"=w802, "Instrument.lvclass"=w804, "S4ACS_GUI in"=w803) -> ("error out"=w784:errorcluster, "S4ACS_GUI out"=w787:refnum<class "S4GUI.lvclass">)  [unwired: 7 in]
          n292 = Select(t=w793, s=w794, f=w788) -> (s? t:f=w785:u32)
          n293 = call-dynamic "Write Acq_state.vi"("error in (no error)"=w784, "Acq_state"=w785, "Acquisition in"=w782) -> ("error out"=w783:errorcluster, "Acquisition out"=w786:refnum<class "Acquisition.lvclass">)  [unwired: 7 in]
        }
        frame 308 {
          n294 = call-dynamic "Read Sync Box.lvclass.vi"("error in (no error)"=w820, "SPARC4_AC in"=w821) -> ("error out"=w810:errorcluster, "Sync Box.lvclass"=w812:refnum<class "Sync Box.lvclass">, "SPARC4_AC out"=w823:refnum<class "S4GUI.lvclass">)  [unwired: 7 in]
          n295 = call "Read connection.vi"("error in (no error)"=w810, "Server in"=w812) -> ("error out"=w809:errorcluster, "connection"=w808:bool, "Server out"=w811:refnum<class "Sync Box.lvclass">)  [unwired: 7 in]
          n296 = case shown="False" w808 {
            tunnel: [w829 w838] -> w824
            tunnel: [w828 w837] -> w822
            tunnel: w819 -> [w827 w836]
            tunnel: [w825 w835] -> w815
            tunnel: w811 -> [w829 w831]
            tunnel: w809 -> [w828 w830]
            frame False {
              # "SyncBox not connected: skip SyncBox trigger"
              n297 = Increment(x=w827) -> (x+1=w826:u32)
              n298 = Increment(x=w826) -> (x+1=w825:u32)
            }
            frame True {
              # "SyncBox connected: performs SyncBox trigger"
              n299 = call-dynamic "Read busy.vi"("error in (no error)"=w830, "Sync Box in"=w831) -> ("error out"=w833:errorcluster, "busy"=w832:bool, "Sync Box out"=w834:refnum<class "Sync Box.lvclass">)  [unwired: 7 in]
              n300 = case shown="False" w832 {
                tunnel: w833 -> [w858 w860]
                tunnel: [w840 w861] -> w838
                tunnel: [w839 w860] -> w837
                tunnel: w836 -> [w848 w859]
                tunnel: w834 -> [w847 w861]
                tunnel: [w844 w859] -> w835
                frame False {
                  # "Sinaliza que SyncBox\nestá ocupado."
                  # "Dispara o comando para o dispositivo corrente."
                  # "envia comando TRIGGER para o SyncBox"
                  n301 = call-dynamic "Read Trigger.lvclass.vi"("error in (no error)"=w858, "Sync Box in"=w847) -> ("error out"=w853:errorcluster, "Trigger.lvclass"=w852:refnum<class "Trigger.lvclass">, "Sync Box out"=w857:refnum<class "Sync Box.lvclass">)  [unwired: 7 in]
                  n302 = call-dynamic "Read State Machine.vi"("error in (no error)"=w853, "Device in"=w852) -> ("error out"=w854:errorcluster, "State Machine.lvclass"=w856:refnum<class "State Machine.lvclass">, "Device out"=w850:refnum<class "Trigger.lvclass">)  [unwired: 7 in]
                  n303 = call "Next State.vi"("error in (no error)"=w854, "New_State"=30, "State Machine in"=w856) -> ("error out"=w845:errorcluster, "State Machine out"=w846:refnum<class "State Machine.lvclass">)  [unwired: 7 in]
                  n304 = call-dynamic "Write State Machine.vi"("error in (no error)"=w845, "State Machine.lvclass"=w846, "Device in"=w850) -> ("error out"=w849:errorcluster, "Device out"=w851:refnum<class "Trigger.lvclass">)  [unwired: 7 in]
                  n305 = call-dynamic "Write Trigger.lvclass.vi"("error in (no error)"=w849, "Trigger.lvclass"=w851, "Sync Box in"=w857) -> ("error out"=w842:errorcluster, "Sync Box out"=w843:refnum<class "Sync Box.lvclass">)  [unwired: 7 in]
                  n306 = Increment(x=w848) -> (x+1=w844:u32)
                  n307 = call-dynamic "Write busy.vi"("error in (no error)"=w842, "busy"=TRUE, "Sync Box in"=w843) -> ("error out"=w839:errorcluster, "Sync Box out"=w840:refnum<class "Sync Box.lvclass">)  [unwired: 7 in]
                }
                frame True {
                }
              }
            }
          }
          n308 = call-dynamic "Write Sync Box.lvclass.vi"("error in (no error)"=w822, "Sync Box.lvclass"=w824, "SPARC4_AC in"=w823) -> ("error out"=w816:errorcluster, "SPARC4_AC out"=w818:refnum<class "S4GUI.lvclass">)  [unwired: 7 in]
          n309 = call-dynamic "Write Acq_state.vi"("error in (no error)"=w816, "Acq_state"=w815, "Acquisition in"=w814) -> ("error out"=w813:errorcluster, "Acquisition out"=w817:refnum<class "Acquisition.lvclass">)  [unwired: 7 in]
        }
        frame 309 {
          # "Espera terminar a execução do comando atual \nantes de ir ao proximo passo da Observação."
          n310 = call-dynamic "Read Sync Box.lvclass.vi"("error in (no error)"=w884, "SPARC4_AC in"=w885) -> ("error out"=w888:errorcluster, "Sync Box.lvclass"=w889:refnum<class "Sync Box.lvclass">, "SPARC4_AC out"=w886:refnum<class "S4GUI.lvclass">)  [unwired: 7 in]
          n311 = call-dynamic "Read Trigger.lvclass.vi"("error in (no error)"=w888, "Sync Box in"=w889) -> ("error out"=w883:errorcluster, "Trigger.lvclass"=w882:refnum<class "Trigger.lvclass">, "Sync Box out"=w887:refnum<class "Sync Box.lvclass">)  [unwired: 7 in]
          n312 = call-dynamic "Read State Machine.vi"("error in (no error)"=w883, "Device in"=w882) -> ("error out"=w876:errorcluster, "State Machine.lvclass"=w878:refnum<class "State Machine.lvclass">, "Device out"=w880:refnum<class "Trigger.lvclass">)  [unwired: 7 in]
          n313 = call-dynamic "Read State.vi"("error in (no error)"=w876, "State Machine in"=w878) -> ("error out"=w875:errorcluster, "State"=w874:i32, "State Machine out"=w877:refnum<class "State Machine.lvclass">)  [unwired: 7 in]
          n314 = Equal To 0?(x=w874) -> (x = 0?=w868:bool)
          n315 = call-dynamic "Write State Machine.vi"("error in (no error)"=w875, "State Machine.lvclass"=w877, "Device in"=w880) -> ("error out"=w879:errorcluster, "Device out"=w881:refnum<class "Trigger.lvclass">)  [unwired: 7 in]
          n316 = call-dynamic "Write Trigger.lvclass.vi"("error in (no error)"=w879, "Trigger.lvclass"=w881, "Sync Box in"=w887) -> ("error out"=w866:errorcluster, "Sync Box out"=w867:refnum<class "Sync Box.lvclass">)  [unwired: 7 in]
          n317 = case shown="True" w868 {
            tunnel: w873 -> [w890 w899]
            tunnel: w867 -> [w892 w898]
            tunnel: w866 -> [w891 w897]
            tunnel: [w891 w896] -> w865
            tunnel: [w892 w895] -> w864
            tunnel: [w890 w893] -> w863
            frame False {
            }
            frame True {
              # "Sinaliza que SyncBox\nestá livre."
              n318 = call-dynamic "Write busy.vi"("error in (no error)"=w897, "busy"=FALSE, "Sync Box in"=w898) -> ("error out"=w896:errorcluster, "Sync Box out"=w895:refnum<class "Sync Box.lvclass">)  [unwired: 7 in]
              n319 = Increment(x=w899) -> (x+1=w893:u32)
            }
          }
          n320 = call-dynamic "Write Sync Box.lvclass.vi"("error in (no error)"=w865, "Sync Box.lvclass"=w864, "SPARC4_AC in"=w886) -> ("error out"=w871:errorcluster, "SPARC4_AC out"=w872:refnum<class "S4GUI.lvclass">)  [unwired: 7 in]
          n321 = call-dynamic "Write Acq_state.vi"("error in (no error)"=w871, "Acq_state"=w863, "Acquisition in"=w862) -> ("error out"=w869:errorcluster, "Acquisition out"=w870:refnum<class "Acquisition.lvclass">)  [unwired: 7 in]
        }
        frame 310 {
          # "Espera terminar a execução do comando atual \nantes de ir ao proximo passo da Observação."
          n322 = call-dynamic "Read Channel.vi"("error in (no error)"=w906, "Acquisition in"=w907) -> ("error out"=w920:errorcluster, "Channel.lvclass"=w919:refnum<class "Channel.lvclass">, "Acquisition out"=w921:refnum<class "Acquisition.lvclass">)  [unwired: 7 in]
          n323 = call-dynamic "Read State Machine.vi"("error in (no error)"=w920, "Device in"=w919) -> ("error out"=w913:errorcluster, "State Machine.lvclass"=w915:refnum<class "State Machine.lvclass">, "Device out"=w917:refnum<class "Channel.lvclass">)  [unwired: 7 in]
          n324 = call-dynamic "Read State.vi"("error in (no error)"=w913, "State Machine in"=w915) -> ("error out"=w912:errorcluster, "State"=w910:i32, "State Machine out"=w914:refnum<class "State Machine.lvclass">)  [unwired: 7 in]
          n325 = call-dynamic "Write State Machine.vi"("error in (no error)"=w912, "State Machine.lvclass"=w914, "Device in"=w917) -> ("error out"=w916:errorcluster, "Device out"=w918:refnum<class "Channel.lvclass">)  [unwired: 7 in]
          n326 = Equal To 0?(x=w910) -> (x = 0?=w911:bool)
          n327 = call-dynamic "Write Channel.vi"("error in (no error)"=w916, "Channel.lvclass"=w918, "Acquisition in"=w921) -> ("error out"=w903:errorcluster, "Acquisition out"=w905:refnum<class "Acquisition.lvclass">)  [unwired: 7 in]
          n328 = Select(t=u32 301, s=w911, f=w909) -> (s? t:f=w904:u32)
          n329 = call-dynamic "Write Acq_state.vi"("error in (no error)"=w903, "Acq_state"=w904, "Acquisition in"=w905) -> ("error out"=w900:errorcluster, "Acquisition out"=w901:refnum<class "Acquisition.lvclass">)  [unwired: 7 in]
        }
        frame 311 {
          n330 = call-dynamic "Read Channel.vi"("error in (no error)"=w938, "Acquisition in"=w937) -> ("error out"=w936:errorcluster, "Channel.lvclass"=w935:refnum<class "Channel.lvclass">, "Acquisition out"=w922:refnum<class "Acquisition.lvclass">)  [unwired: 7 in]
          n331 = call-dynamic "Read ciclos.vi"("error in (no error)"=w936, "Channel in"=w935) -> ("error out"=w932:errorcluster, "ciclos"=w934:u32, "Channel out"=w923:refnum<class "Channel.lvclass">)  [unwired: 7 in]
          n332 = Decrement(x=w934) -> (x-1=w939:u32)
          n333 = Greater Than 0?(x=w939) -> (x > 0?=w943:bool)
          n334 = case shown="True" w943 {
            selector: w943 -> [w945 w947]
            tunnel: w939 -> [_ w946]
            tunnel: [w945 w947] -> w942
            tunnel: [u32 0 w946] -> w928
            frame False {
            }
            frame True {
            }
          }
          n335 = call-dynamic "Write ciclos.vi"("error in (no error)"=w932, "ciclos"=w928, "Channel in"=w923) -> ("error out"=w930:errorcluster, "Channel out"=w929:refnum<class "Channel.lvclass">)  [unwired: 7 in]
          n336 = Select(t=u32 301, s=w942, f=u32 0) -> (s? t:f=w933:u32)
          n337 = call-dynamic "Write Channel.vi"("error in (no error)"=w930, "Channel.lvclass"=w929, "Acquisition in"=w922) -> ("error out"=w926:errorcluster, "Acquisition out"=w927:refnum<class "Acquisition.lvclass">)  [unwired: 7 in]
          n338 = call-dynamic "Write Acq_state.vi"("error in (no error)"=w926, "Acq_state"=w933, "Acquisition in"=w927) -> ("error out"=w924:errorcluster, "Acquisition out"=w925:refnum<class "Acquisition.lvclass">)  [unwired: 7 in]
        }
        frame 321 {
          n339 = call-dynamic "Read Sync Box.lvclass.vi"("error in (no error)"=w960, "SPARC4_AC in"=w961) -> ("error out"=w950:errorcluster, "Sync Box.lvclass"=w951:refnum<class "Sync Box.lvclass">, "SPARC4_AC out"=w963:refnum<class "S4GUI.lvclass">)  [unwired: 7 in]
          n340 = call "Read connection.vi"("error in (no error)"=w950, "Server in"=w951) -> ("error out"=w949:errorcluster, "connection"=w948:bool, "Server out"=w952:refnum<class "Sync Box.lvclass">)  [unwired: 7 in]
          n341 = case shown="True" w948 {
            tunnel: [w969 w978] -> w964
            tunnel: [w968 w977] -> w962
            tunnel: w959 -> [w967 w976]
            tunnel: [w965 w975] -> w955
            tunnel: w952 -> [w969 w974]
            tunnel: w949 -> [w968 w973]
            frame False {
              # "SyncBox not connected: skip SyncBox configuration"
              n342 = Increment(x=w967) -> (x+1=w966:u32)
              n343 = Increment(x=w966) -> (x+1=w965:u32)
            }
            frame True {
              # "SyncBox connected: Performs  SyncBox configuration"
              n344 = call-dynamic "Read busy.vi"("error in (no error)"=w973, "Sync Box in"=w974) -> ("error out"=w970:errorcluster, "busy"=w972:bool, "Sync Box out"=w971:refnum<class "Sync Box.lvclass">)  [unwired: 7 in]
              n345 = case shown="False" w972 {
                tunnel: [w982 w1004] -> w978
                tunnel: [w980 w1003] -> w977
                tunnel: w976 -> [w992 w1002]
                tunnel: [w986 w1002] -> w975
                tunnel: w971 -> [w985 w1004]
                tunnel: w970 -> [w984 w1003]
                frame False {
                  # "configura delays do syncBox"
                  # "Dispara o comando para o dispositivo corrente."
                  n346 = call-dynamic "Read Trigger.lvclass.vi"("error in (no error)"=w984, "Sync Box in"=w985) -> ("error out"=w997:errorcluster, "Trigger.lvclass"=w996:refnum<class "Trigger.lvclass">, "Sync Box out"=w1001:refnum<class "Sync Box.lvclass">)  [unwired: 7 in]
                  n347 = call-dynamic "Read State Machine.vi"("error in (no error)"=w997, "Device in"=w996) -> ("error out"=w998:errorcluster, "State Machine.lvclass"=w1000:refnum<class "State Machine.lvclass">, "Device out"=w994:refnum<class "Trigger.lvclass">)  [unwired: 7 in]
                  n348 = call "Next State.vi"("error in (no error)"=w998, "New_State"=10, "State Machine in"=w1000) -> ("error out"=w988:errorcluster, "State Machine out"=w990:refnum<class "State Machine.lvclass">)  [unwired: 7 in]
                  n349 = call-dynamic "Write Timer.vi"("error in (no error)"=w988, "Timer"=u32 5, "State Machine in"=w990) -> ("error out"=w987:errorcluster, "State Machine out"=w989:refnum<class "State Machine.lvclass">)  [unwired: 7 in]
                  n350 = call-dynamic "Write State Machine.vi"("error in (no error)"=w987, "State Machine.lvclass"=w989, "Device in"=w994) -> ("error out"=w993:errorcluster, "Device out"=w995:refnum<class "Trigger.lvclass">)  [unwired: 7 in]
                  n351 = call-dynamic "Write Trigger.lvclass.vi"("error in (no error)"=w993, "Trigger.lvclass"=w995, "Sync Box in"=w1001) -> ("error out"=w981:errorcluster, "Sync Box out"=w983:refnum<class "Sync Box.lvclass">)  [unwired: 7 in]
                  n352 = Increment(x=w992) -> (x+1=w986:u32)
                  n353 = call-dynamic "Write busy.vi"("error in (no error)"=w981, "busy"=TRUE, "Sync Box in"=w983) -> ("error out"=w980:errorcluster, "Sync Box out"=w982:refnum<class "Sync Box.lvclass">)  [unwired: 7 in]
                }
                frame True {
                }
              }
            }
          }
          n354 = call-dynamic "Write Sync Box.lvclass.vi"("error in (no error)"=w962, "Sync Box.lvclass"=w964, "SPARC4_AC in"=w963) -> ("error out"=w956:errorcluster, "SPARC4_AC out"=w958:refnum<class "S4GUI.lvclass">)  [unwired: 7 in]
          n355 = call-dynamic "Write Acq_state.vi"("error in (no error)"=w956, "Acq_state"=w955, "Acquisition in"=w954) -> ("error out"=w953:errorcluster, "Acquisition out"=w957:refnum<class "Acquisition.lvclass">)  [unwired: 7 in]
        }
        frame 322 {
          # "Espera terminar a execução do comando atual \nantes de ir ao proximo passo da Observação."
          n356 = call-dynamic "Read Sync Box.lvclass.vi"("error in (no error)"=w1027, "SPARC4_AC in"=w1028) -> ("error out"=w1031:errorcluster, "Sync Box.lvclass"=w1032:refnum<class "Sync Box.lvclass">, "SPARC4_AC out"=w1029:refnum<class "S4GUI.lvclass">)  [unwired: 7 in]
          n357 = call-dynamic "Read Trigger.lvclass.vi"("error in (no error)"=w1031, "Sync Box in"=w1032) -> ("error out"=w1026:errorcluster, "Trigger.lvclass"=w1025:refnum<class "Trigger.lvclass">, "Sync Box out"=w1030:refnum<class "Sync Box.lvclass">)  [unwired: 7 in]
          n358 = call-dynamic "Read State Machine.vi"("error in (no error)"=w1026, "Device in"=w1025) -> ("error out"=w1019:errorcluster, "State Machine.lvclass"=w1021:refnum<class "State Machine.lvclass">, "Device out"=w1023:refnum<class "Trigger.lvclass">)  [unwired: 7 in]
          n359 = call-dynamic "Read State.vi"("error in (no error)"=w1019, "State Machine in"=w1021) -> ("error out"=w1018:errorcluster, "State"=w1017:i32, "State Machine out"=w1020:refnum<class "State Machine.lvclass">)  [unwired: 7 in]
          n360 = Equal To 0?(x=w1017) -> (x = 0?=w1005:bool)
          n361 = call-dynamic "Write State Machine.vi"("error in (no error)"=w1018, "State Machine.lvclass"=w1020, "Device in"=w1023) -> ("error out"=w1022:errorcluster, "Device out"=w1024:refnum<class "Trigger.lvclass">)  [unwired: 7 in]
          n362 = call-dynamic "Write Trigger.lvclass.vi"("error in (no error)"=w1022, "Trigger.lvclass"=w1024, "Sync Box in"=w1030) -> ("error out"=w1007:errorcluster, "Sync Box out"=w1009:refnum<class "Sync Box.lvclass">)  [unwired: 7 in]
          n363 = case shown="True" w1005 {
            tunnel: w1016 -> [w1035 w1042]
            tunnel: [w1035 w1041] -> w1010
            tunnel: [w1034 w1039] -> w1008
            tunnel: w1009 -> [w1034 w1040]
            tunnel: [w1033 w1037] -> w1006
            tunnel: w1007 -> [w1033 w1038]
            frame False {
            }
            frame True {
              n364 = call-dynamic "Write busy.vi"("error in (no error)"=w1038, "busy"=FALSE, "Sync Box in"=w1040) -> ("error out"=w1037:errorcluster, "Sync Box out"=w1039:refnum<class "Sync Box.lvclass">)  [unwired: 7 in]
              n365 = Increment(x=w1042) -> (x+1=w1041:u32)
            }
          }
          n366 = call-dynamic "Write Sync Box.lvclass.vi"("error in (no error)"=w1006, "Sync Box.lvclass"=w1008, "SPARC4_AC in"=w1029) -> ("error out"=w1013:errorcluster, "SPARC4_AC out"=w1015:refnum<class "S4GUI.lvclass">)  [unwired: 7 in]
          n367 = call-dynamic "Write Acq_state.vi"("error in (no error)"=w1013, "Acq_state"=w1010, "Acquisition in"=w1011) -> ("error out"=w1012:errorcluster, "Acquisition out"=w1014:refnum<class "Acquisition.lvclass">)  [unwired: 7 in]
        }
        frame 323 {
          # "Dispara o comando para o dispositivo corrente."
          n368 = call-dynamic "Read Channel.vi"("error in (no error)"=w1049, "Acquisition in"=w1050) -> ("error out"=w1061:errorcluster, "Channel.lvclass"=w1060:refnum<class "Channel.lvclass">, "Acquisition out"=w1065:refnum<class "Acquisition.lvclass">)  [unwired: 7 in]
          n369 = call-dynamic "Read State Machine.vi"("error in (no error)"=w1061, "Device in"=w1060) -> ("error out"=w1062:errorcluster, "State Machine.lvclass"=w1064:refnum<class "State Machine.lvclass">, "Device out"=w1058:refnum<class "Channel.lvclass">)  [unwired: 7 in]
          n370 = call "Next State.vi"("error in (no error)"=w1062, "New_State"=50, "State Machine in"=w1064) -> ("error out"=w1052:errorcluster, "State Machine out"=w1054:refnum<class "State Machine.lvclass">)  [unwired: 7 in]
          n371 = call-dynamic "Write Timer.vi"("error in (no error)"=w1052, "Timer"=u32 2, "State Machine in"=w1054) -> ("error out"=w1051:errorcluster, "State Machine out"=w1053:refnum<class "State Machine.lvclass">)  [unwired: 7 in]
          n372 = call-dynamic "Write State Machine.vi"("error in (no error)"=w1051, "State Machine.lvclass"=w1053, "Device in"=w1058) -> ("error out"=w1057:errorcluster, "Device out"=w1059:refnum<class "Channel.lvclass">)  [unwired: 7 in]
          n373 = Increment(x=w1056) -> (x+1=w1046:u32)
          n374 = call-dynamic "Write Channel.vi"("error in (no error)"=w1057, "Channel.lvclass"=w1059, "Acquisition in"=w1065) -> ("error out"=w1045:errorcluster, "Acquisition out"=w1047:refnum<class "Acquisition.lvclass">)  [unwired: 7 in]
          n375 = call-dynamic "Write Acq_state.vi"("error in (no error)"=w1045, "Acq_state"=w1046, "Acquisition in"=w1047) -> ("error out"=w1043:errorcluster, "Acquisition out"=w1048:refnum<class "Acquisition.lvclass">)  [unwired: 7 in]
        }
        frame 324 {
          n376 = call-dynamic "Read Sync Box.lvclass.vi"("error in (no error)"=w1078, "SPARC4_AC in"=w1079) -> ("error out"=w1069:errorcluster, "Sync Box.lvclass"=w1070:refnum<class "Sync Box.lvclass">, "SPARC4_AC out"=w1081:refnum<class "S4GUI.lvclass">)  [unwired: 7 in]
          n377 = call "Read connection.vi"("error in (no error)"=w1069, "Server in"=w1070) -> ("error out"=w1068:errorcluster, "connection"=w1066:bool, "Server out"=w1067:refnum<class "Sync Box.lvclass">)  [unwired: 7 in]
          n378 = case shown="True" w1066 {
            tunnel: [w1087 w1096] -> w1082
            tunnel: [w1086 w1095] -> w1080
            tunnel: w1077 -> [w1085 w1094]
            tunnel: [w1083 w1090] -> w1075
            tunnel: w1068 -> [w1086 w1089]
            tunnel: w1067 -> [w1087 w1088]
            frame False {
              # "SyncBox not connected: skip SyncBox trigger"
              n379 = Increment(x=w1085) -> (x+1=w1084:u32)
              n380 = Increment(x=w1084) -> (x+1=w1083:u32)
            }
            frame True {
              # "SyncBox connected: Performs  SyncBox trigger"
              n381 = call-dynamic "Read busy.vi"("error in (no error)"=w1089, "Sync Box in"=w1088) -> ("error out"=w1091:errorcluster, "busy"=w1093:bool, "Sync Box out"=w1092:refnum<class "Sync Box.lvclass">)  [unwired: 7 in]
              n382 = case shown="False" w1093 {
                tunnel: w1091 -> [w1116 w1118]
                tunnel: [w1100 w1119] -> w1096
                tunnel: [w1098 w1118] -> w1095
                tunnel: w1094 -> [w1106 w1117]
                tunnel: [w1105 w1117] -> w1090
                tunnel: w1092 -> [w1104 w1119]
                frame False {
                  # "configura o TRIGGER e dispara o SyncBox"
                  # "Dispara o comando para o dispositivo corrente."
                  n383 = call-dynamic "Read Trigger.lvclass.vi"("error in (no error)"=w1116, "Sync Box in"=w1104) -> ("error out"=w1111:errorcluster, "Trigger.lvclass"=w1110:refnum<class "Trigger.lvclass">, "Sync Box out"=w1115:refnum<class "Sync Box.lvclass">)  [unwired: 7 in]
                  n384 = call-dynamic "Read State Machine.vi"("error in (no error)"=w1111, "Device in"=w1110) -> ("error out"=w1112:errorcluster, "State Machine.lvclass"=w1114:refnum<class "State Machine.lvclass">, "Device out"=w1108:refnum<class "Trigger.lvclass">)  [unwired: 7 in]
                  n385 = call "Next State.vi"("error in (no error)"=w1112, "New_State"=30, "State Machine in"=w1114) -> ("error out"=w1102:errorcluster, "State Machine out"=w1103:refnum<class "State Machine.lvclass">)  [unwired: 7 in]
                  n386 = call-dynamic "Write State Machine.vi"("error in (no error)"=w1102, "State Machine.lvclass"=w1103, "Device in"=w1108) -> ("error out"=w1107:errorcluster, "Device out"=w1109:refnum<class "Trigger.lvclass">)  [unwired: 7 in]
                  n387 = Increment(x=w1106) -> (x+1=w1105:u32)
                  n388 = call-dynamic "Write Trigger.lvclass.vi"("error in (no error)"=w1107, "Trigger.lvclass"=w1109, "Sync Box in"=w1115) -> ("error out"=w1099:errorcluster, "Sync Box out"=w1101:refnum<class "Sync Box.lvclass">)  [unwired: 7 in]
                  n389 = call-dynamic "Write busy.vi"("error in (no error)"=w1099, "busy"=TRUE, "Sync Box in"=w1101) -> ("error out"=w1098:errorcluster, "Sync Box out"=w1100:refnum<class "Sync Box.lvclass">)  [unwired: 7 in]
                }
                frame True {
                }
              }
            }
          }
          n390 = call-dynamic "Write Sync Box.lvclass.vi"("error in (no error)"=w1080, "Sync Box.lvclass"=w1082, "SPARC4_AC in"=w1081) -> ("error out"=w1074:errorcluster, "SPARC4_AC out"=w1076:refnum<class "S4GUI.lvclass">)  [unwired: 7 in]
          n391 = call-dynamic "Write Acq_state.vi"("error in (no error)"=w1074, "Acq_state"=w1075, "Acquisition in"=w1071) -> ("error out"=w1073:errorcluster, "Acquisition out"=w1072:refnum<class "Acquisition.lvclass">)  [unwired: 7 in]
        }
        frame 325 {
          # "Espera terminar a execução do comando atual \nantes de ir ao proximo passo da Observação."
          n392 = call-dynamic "Read Sync Box.lvclass.vi"("error in (no error)"=w1142, "SPARC4_AC in"=w1143) -> ("error out"=w1146:errorcluster, "Sync Box.lvclass"=w1147:refnum<class "Sync Box.lvclass">, "SPARC4_AC out"=w1144:refnum<class "S4GUI.lvclass">)  [unwired: 7 in]
          n393 = call-dynamic "Read Trigger.lvclass.vi"("error in (no error)"=w1146, "Sync Box in"=w1147) -> ("error out"=w1141:errorcluster, "Trigger.lvclass"=w1140:refnum<class "Trigger.lvclass">, "Sync Box out"=w1145:refnum<class "Sync Box.lvclass">)  [unwired: 7 in]
          n394 = call-dynamic "Read State Machine.vi"("error in (no error)"=w1141, "Device in"=w1140) -> ("error out"=w1134:errorcluster, "State Machine.lvclass"=w1136:refnum<class "State Machine.lvclass">, "Device out"=w1138:refnum<class "Trigger.lvclass">)  [unwired: 7 in]
          n395 = call-dynamic "Read State.vi"("error in (no error)"=w1134, "State Machine in"=w1136) -> ("error out"=w1133:errorcluster, "State"=w1132:i32, "State Machine out"=w1135:refnum<class "State Machine.lvclass">)  [unwired: 7 in]
          n396 = Equal To 0?(x=w1132) -> (x = 0?=w1126:bool)
          n397 = call-dynamic "Write State Machine.vi"("error in (no error)"=w1133, "State Machine.lvclass"=w1135, "Device in"=w1138) -> ("error out"=w1137:errorcluster, "Device out"=w1139:refnum<class "Trigger.lvclass">)  [unwired: 7 in]
          n398 = call-dynamic "Write Trigger.lvclass.vi"("error in (no error)"=w1137, "Trigger.lvclass"=w1139, "Sync Box in"=w1145) -> ("error out"=w1124:errorcluster, "Sync Box out"=w1125:refnum<class "Sync Box.lvclass">)  [unwired: 7 in]
          n399 = case shown="True" w1126 {
            tunnel: w1131 -> [w1148 w1157]
            tunnel: [w1150 w1155] -> w1122
            tunnel: w1125 -> [w1150 w1156]
            tunnel: [w1149 w1153] -> w1123
            tunnel: w1124 -> [w1149 w1154]
            tunnel: [w1148 w1152] -> w1121
            frame False {
            }
            frame True {
              n400 = Increment(x=w1157) -> (x+1=w1152:u32)
              n401 = call-dynamic "Write busy.vi"("error in (no error)"=w1154, "busy"=FALSE, "Sync Box in"=w1156) -> ("error out"=w1153:errorcluster, "Sync Box out"=w1155:refnum<class "Sync Box.lvclass">)  [unwired: 7 in]
            }
          }
          n402 = call-dynamic "Write Sync Box.lvclass.vi"("error in (no error)"=w1123, "Sync Box.lvclass"=w1122, "SPARC4_AC in"=w1144) -> ("error out"=w1129:errorcluster, "SPARC4_AC out"=w1130:refnum<class "S4GUI.lvclass">)  [unwired: 7 in]
          n403 = call-dynamic "Write Acq_state.vi"("error in (no error)"=w1129, "Acq_state"=w1121, "Acquisition in"=w1120) -> ("error out"=w1127:errorcluster, "Acquisition out"=w1128:refnum<class "Acquisition.lvclass">)  [unwired: 7 in]
        }
        frame 326 {
          # "Espera terminar a execução do comando atual \nantes de ir ao proximo passo da Observação."
          n404 = call-dynamic "Read Channel.vi"("error in (no error)"=w1159, "Acquisition in"=w1158) -> ("error out"=w1178:errorcluster, "Channel.lvclass"=w1177:refnum<class "Channel.lvclass">, "Acquisition out"=w1179:refnum<class "Acquisition.lvclass">)  [unwired: 7 in]
          n405 = call-dynamic "Read State Machine.vi"("error in (no error)"=w1178, "Device in"=w1177) -> ("error out"=w1171:errorcluster, "State Machine.lvclass"=w1173:refnum<class "State Machine.lvclass">, "Device out"=w1175:refnum<class "Channel.lvclass">)  [unwired: 7 in]
          n406 = call-dynamic "Read State.vi"("error in (no error)"=w1171, "State Machine in"=w1173) -> ("error out"=w1170:errorcluster, "State"=w1168:i32, "State Machine out"=w1172:refnum<class "State Machine.lvclass">)  [unwired: 7 in]
          n407 = Equal To 0?(x=w1168) -> (x = 0?=w1169:bool)
          n408 = call-dynamic "Write State Machine.vi"("error in (no error)"=w1170, "State Machine.lvclass"=w1172, "Device in"=w1175) -> ("error out"=w1174:errorcluster, "Device out"=w1176:refnum<class "Channel.lvclass">)  [unwired: 7 in]
          n409 = call-dynamic "Write Channel.vi"("error in (no error)"=w1174, "Channel.lvclass"=w1176, "Acquisition in"=w1179) -> ("error out"=w1161:errorcluster, "Acquisition out"=w1162:refnum<class "Acquisition.lvclass">)  [unwired: 7 in]
          n410 = Increment(x=w1167) -> (x+1=w1166:u32)
          n411 = Select(t=w1166, s=w1169, f=w1167) -> (s? t:f=w1164:u32)
          n412 = call-dynamic "Write Acq_state.vi"("error in (no error)"=w1161, "Acq_state"=w1164, "Acquisition in"=w1162) -> ("error out"=w1163:errorcluster, "Acquisition out"=w1165:refnum<class "Acquisition.lvclass">)  [unwired: 7 in]
        }
        frame 327 {
          n413 = call-dynamic "Read Channel.vi"("error in (no error)"=w1195, "Acquisition in"=w1196) -> ("error out"=w1193:errorcluster, "Channel.lvclass"=w1194:refnum<class "Channel.lvclass">, "Acquisition out"=w1189:refnum<class "Acquisition.lvclass">)  [unwired: 7 in]
          n414 = call-dynamic "Read ciclos.vi"("error in (no error)"=w1193, "Channel in"=w1194) -> ("error out"=w1184:errorcluster, "ciclos"=w1192:u32, "Channel out"=w1185:refnum<class "Channel.lvclass">)  [unwired: 7 in]
          n415 = Decrement(x=w1192) -> (x-1=w1197:u32)
          n416 = Greater Than 0?(x=w1197) -> (x > 0?=w1201:bool)
          n417 = case shown="True" w1201 {
            selector: w1201 -> [w1203 w1205]
            tunnel: w1197 -> [_ w1204]
            tunnel: [w1203 w1205] -> w1200
            tunnel: [u32 0 w1204] -> w1190
            frame False {
            }
            frame True {
            }
          }
          n418 = call-dynamic "Write ciclos.vi"("error in (no error)"=w1184, "ciclos"=w1190, "Channel in"=w1185) -> ("error out"=w1183:errorcluster, "Channel out"=w1186:refnum<class "Channel.lvclass">)  [unwired: 7 in]
          n419 = call-dynamic "Write Channel.vi"("error in (no error)"=w1183, "Channel.lvclass"=w1186, "Acquisition in"=w1189) -> ("error out"=w1182:errorcluster, "Acquisition out"=w1188:refnum<class "Acquisition.lvclass">)  [unwired: 7 in]
          n420 = Select(t=u32 321, s=w1200, f=u32 0) -> (s? t:f=w1180:u32)
          n421 = call-dynamic "Write Acq_state.vi"("error in (no error)"=w1182, "Acq_state"=w1180, "Acquisition in"=w1188) -> ("error out"=w1181:errorcluster, "Acquisition out"=w1187:refnum<class "Acquisition.lvclass">)  [unwired: 7 in]
        }
        frame 400 {
          # "Estado de \"Pause\": fica parado aqui até o botão START seja pressionado."
        }
      }
    }
    frame Error {
    }
  }
  "error out" <- w5
  "S4ACS_GUI out" <- w3
  "Acquisition.lvclass Out" <- w1
